vi "Module - Page User.vi"() -> ()   [LabVIEW 2020]
uses:
  Control/Cluster - User Information.ctl
  Control/Header - User Access Level.ctl
  Control/Button/Select Option 2.ctl
  Control/State - Module User Management.ctl
  Control/Password Setting Data.ctl
  Control/State - FGV.ctl
  Control/State - eFGV.ctl
  Control/aFGV States - Subpanel.ctl
  Control/User Authorization Info.ctl
  Control/Header - User Management.ctl
  a4231f55-2fe4-47fd-8ff5-63e6bb856ac6.vi
  762b96f1-960b-474f-bf97-e387c57ec164.vi
  Control/State - Directory.ctl
panel:
  in  "Tab Control":T1(tab)
  in  "Filter:":string(combo)="Show All" caption="Select Access Level:"
  in  "Clear Search":bool
  in  "Search Bar":string
  in  "Search By:":T2
  in  "Setting":bool
  in  "Add User":bool
  in  "User Information":T3[](array[typedef])
  in  "Stop":bool
  out "Header":T4
  in  "Search User":string(combo)
  out "Delete Msg":bool
  in  "Config: Access Level":string(combo) caption="Access Level:"
  in  "Password:":string
  in  "Username:":string
  in  "Name:":string
  in  "Config: Update":bool
  in  "Back 1":bool
  in  "Config: All Page":i32(listbox) caption="All Page"
  in  "Config: Accessible Page":i32(listbox) caption="Accessible Page"
  in  "Config: Add Page":bool
  in  "Config: Delete Page":bool
  in  "Config: Reset Page":bool
  in  "Back 2":bool
  in  "Manage: Access Level":string(combo)="Admin" caption="Access Level:"
  in  "Manage: All Page":i32(listbox) caption="All Page"
  in  "Manage: Accessible Page":i32(listbox) caption="Accessible Page"
  in  "Manage: Delete Page":bool
  in  "Manage: Add Page":bool
  in  "Header - User Access Level":T5
  in  "Staff Id":string caption="Staff Id:"
  in  "New Name:":string caption="Name:"
  in  "New Username:":string caption="Username:"
  in  "New Password:":string caption="Password:"
  in  "New Access Level:":string(combo) caption="Access Level:"
  in  "Re-Type Password:":string caption="Password:"
  in  "Create User":bool
  in  "Cancel Create User":bool
  in  "Back 3":bool
  in  "User Information T":i32(listbox) caption="User Information Listbox"
  in  "Access Page T":i32(listbox) caption="User Information Listbox"
  # "Manage User Account"
  # "Configure User Account"
  # "Manage User Access"
  # "Create New User"
  # "Fill up all information"
  # "Data Acquisition System"
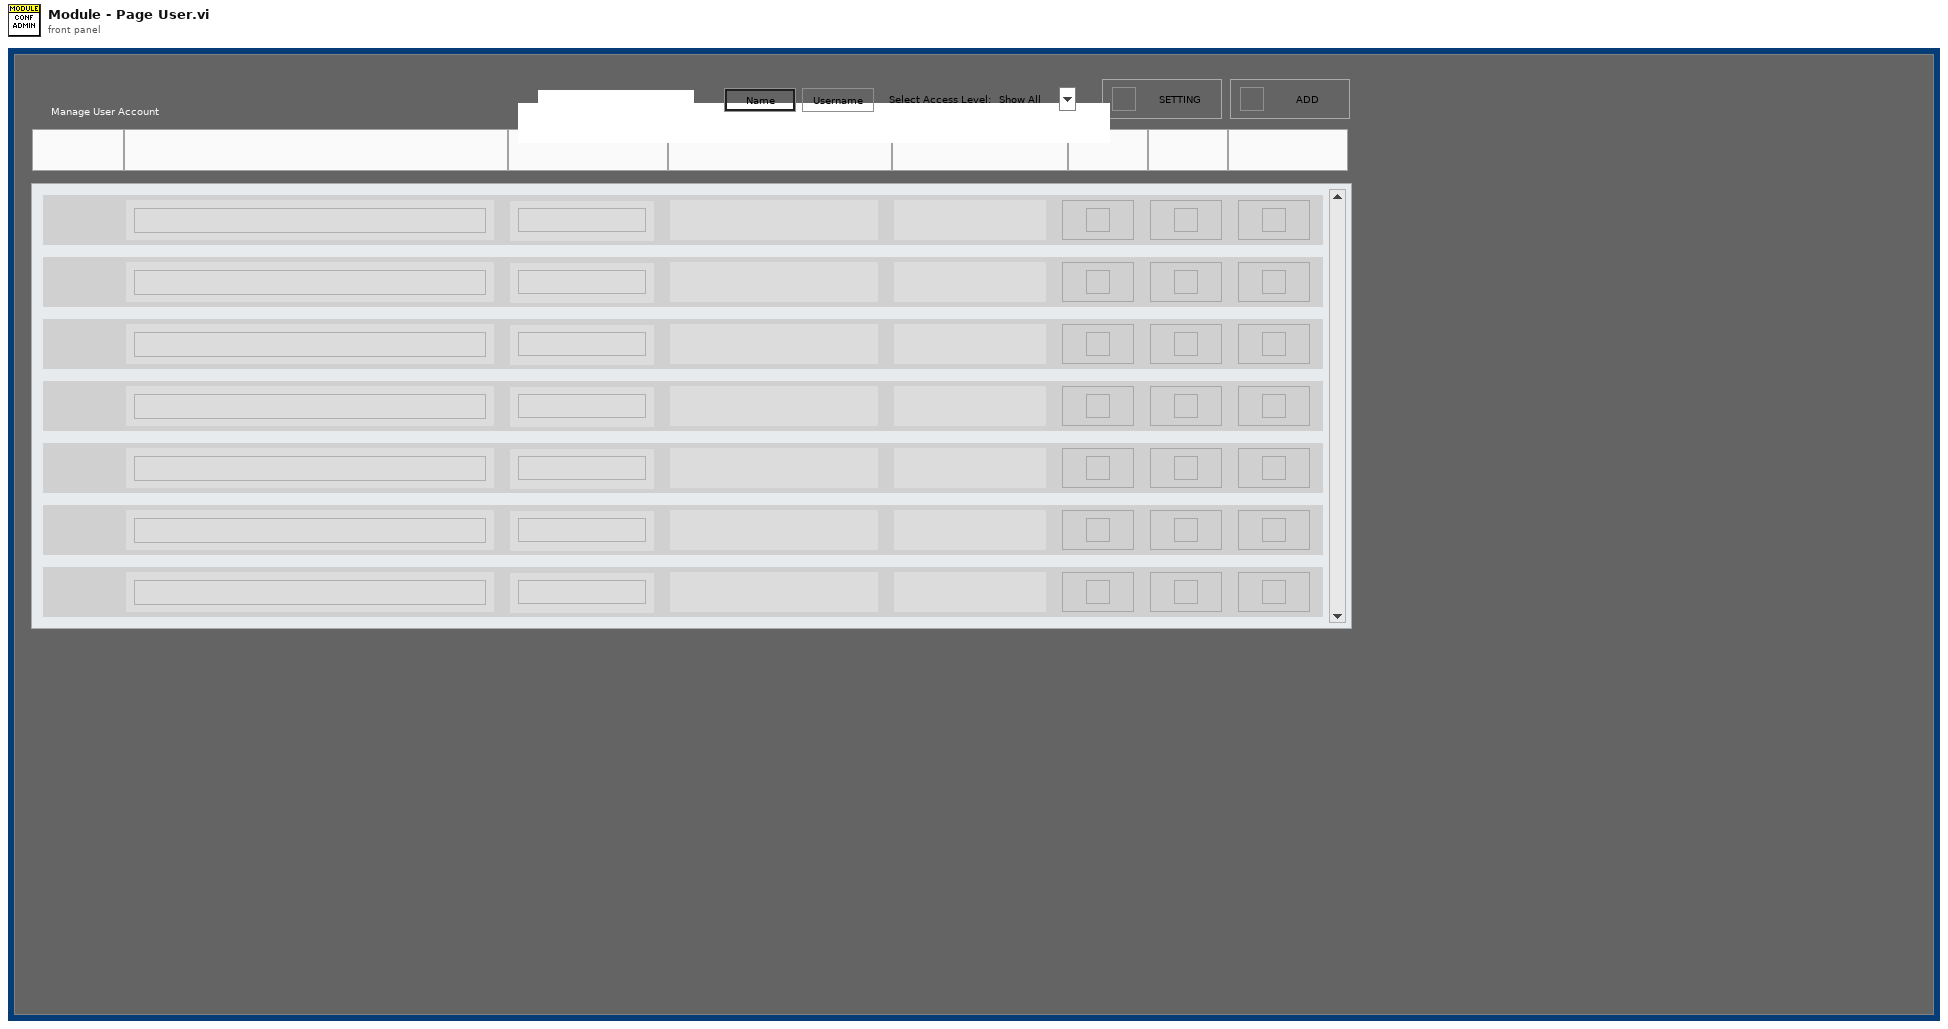
[diagram p1: front panel]
types:
  T1 = enum32{"Table", "Edit User", "Config", "New User", "Preference"}
  T2 = typedef "Select Option 2.ctl" = enum32{"L", "R"}
  T3 = typedef "Cluster - User Information.ctl" = cluster{"Access Level":u16, "Name":string, "Staff ID":string, "Username":string, "Password":string, "Configure":bool, "Status":bool, "Remove":bool}
  T4 = cluster{"Data 1":string, "Data 2":string, "Data 3":string, "Data 4":string, "Data 5":string, "Data 7":string, "Data 8":string, "Data 9":string}
  T5 = typedef "Header - User Access Level.ctl" = enum16{"Admin", "Manager", "Engineer", "Technician"}
  T6 = enum16{"Init", "Init Page", "Register Events", "Load User Access Page", "Load User Authorization Info", "Create Folder Data", "Update Folder Data", "Logout", "Idle", "Query DB Authrorization Info", "Update Authorization Info", "Reset User Access Page", "Add User Access Page", "Remove User Access Page", "Save User Authorization Info", "Search User", "Verify New User", "Create New User", "Update Authrorization Data", "Update Selected User", "Edit User Info", "Check Logged User", "Remove", "Block", "Add Config Access Page", "Remove Config Access Page", "Update Config User Access", "Save Config Access Page", "Save Password Settg", "Exit"}
  T7 = typedef "Password Setting Data.ctl" = cluster{"Length":i32, "Special Char":i32, "Numeric":i32, "Alphabet":i32}
  T8 = cluster{"Table":string[][], "Selected Row":i32, "Process":string, "Password Setting":T7, "Column Header Strings":string[], "Initialized Row":string[], "User Info":cluster{"Name":string, "Username":string, "Password":string, "Level":string, "Block":string, "Show Password":bool}, "Path User Info":path, "Path User Access":path, "Update User":bool, "Old Username":string, "Username Updated?":bool, "User Information":cluster{"All":T3[], "Filtered":T3[]}}
  T9 = typedef "State - Module User Management.ctl" = enum16{"Init", "Init Page", "Register Events", "Load User Access Page", "Load User Authorization Info", "Create Folder Data", "Update Folder Data", "Logout", "Idle", "Query DB Authrorization Info", "Update Authorization Info", "Reset User Access Page", "Add User Access Page", "Remove User Access Page", "Save User Authorization Info", "Search User", "Verify New User", "Create New User", "Update Authrorization Data", "Update Selected User", "Edit User Info", "Check Logged User", "Remove", "Block", "Add Config Access Page", "Remove Config Access Page", "Update Config User Access", "Save Config Access Page", "Save Password Settg", "Exit"}
  T10 = typedef "State - FGV.ctl" = enum16{"Write", "Read"}
  T11 = typedef "aFGV States - Subpanel.ctl" = enum16{"Init", "Get VI Name", "Update", "Exit"}
  T12 = typedef "State - eFGV.ctl" = enum16{"Init", "Read", "Write", "Exit"}
  T13 = typedef "Header - User Management.ctl" = enum16{"Name", "Staff ID", "Username", "Password", "Access Level", "Status", "Access Page"}
  T14 = enum8{"Enabled", "Disabled", "Disabled and Grayed Out"}
  T15 = enum32{"Table", "Edit User", "Config", "New User"}
  T16 = typedef "State - Directory.ctl" = enum16{"Plant", "Config", "Admin", "Password", "Modules", "Dialog Box", "SubVI", "Setting"}
  T17 = enum16{"open", "replace", "create", "open or create", "replace or create", "replace or create with confirmation"}
  T18 = typedef "Page List Configuration.ctl" = cluster{"HMI Configuration":cluster{"EXE Name":string, "Project Name":string, "Max Page No":i32, "HMI State":enum32{"Invalid", "Standard", "Closed", "Hidden", "Minimized", "Maximized"}, "Version":enum16{"Demo", "User"}, "Check License":bool, "Font Size":u32, "Res: Height":i16, "Res: Width":i16, "License Level":enum16{"Level 1", "Level 2", "Level 3", "Level 4", "Level 5"}, "License Type":enum16{"Free", "Trial", "Subscription", "Perpetual"}}, "All HMI Module":string[], "Default HMI Module":string[], "Page Module":string[], "Page List: Level 1":string[], "Page List: Level 2":string[], "Page List: Level 3":string[], "All RT Module":string[], "Default RT Module":string[], "Acquire Enable Page":string[], "Log Enable Page":string[], "Run Page":string[], "Kill Page":string[], "Button":cluster{"Text":string[], "Tip Strip":string[]}}
  T19 = typedef "License File Parameter.ctl" = cluster{"Expired Time":string, "Computer ID":string, "Product Name":string, "Period":i16, "Activated Time":string, "License Level":enum16{"Level 1", "Level 2", "Level 3", "Level 4", "Level 5"}, "License Type":enum16{"Free", "Trial", "Subscription", "Perpetual"}, "Log Time":string}
  T20 = enum16{"Level 1", "Level 2", "Level 3", "Level 4", "Level 5"}
  T21 = cluster{"Access Level:":string, "List Page":string[]}[]
  T22 = typedef "User Authorization Info.ctl" = cluster{"Name":string, "Username":string, "Password":string, "Access Level:":string, "Block":string, "List Page":string[]}
  T23 = cluster{"Access Level":bool, "Name":bool, "Staff ID":bool, "Username":bool, "Password":bool, "Configure":bool, "Status":bool, "Remove":bool}
  T24 = enum32{"invalid app kind", "Development System", "Run Time System", "Student Edition", "Embedded LabVIEW", "Evaluation", "Custom"}
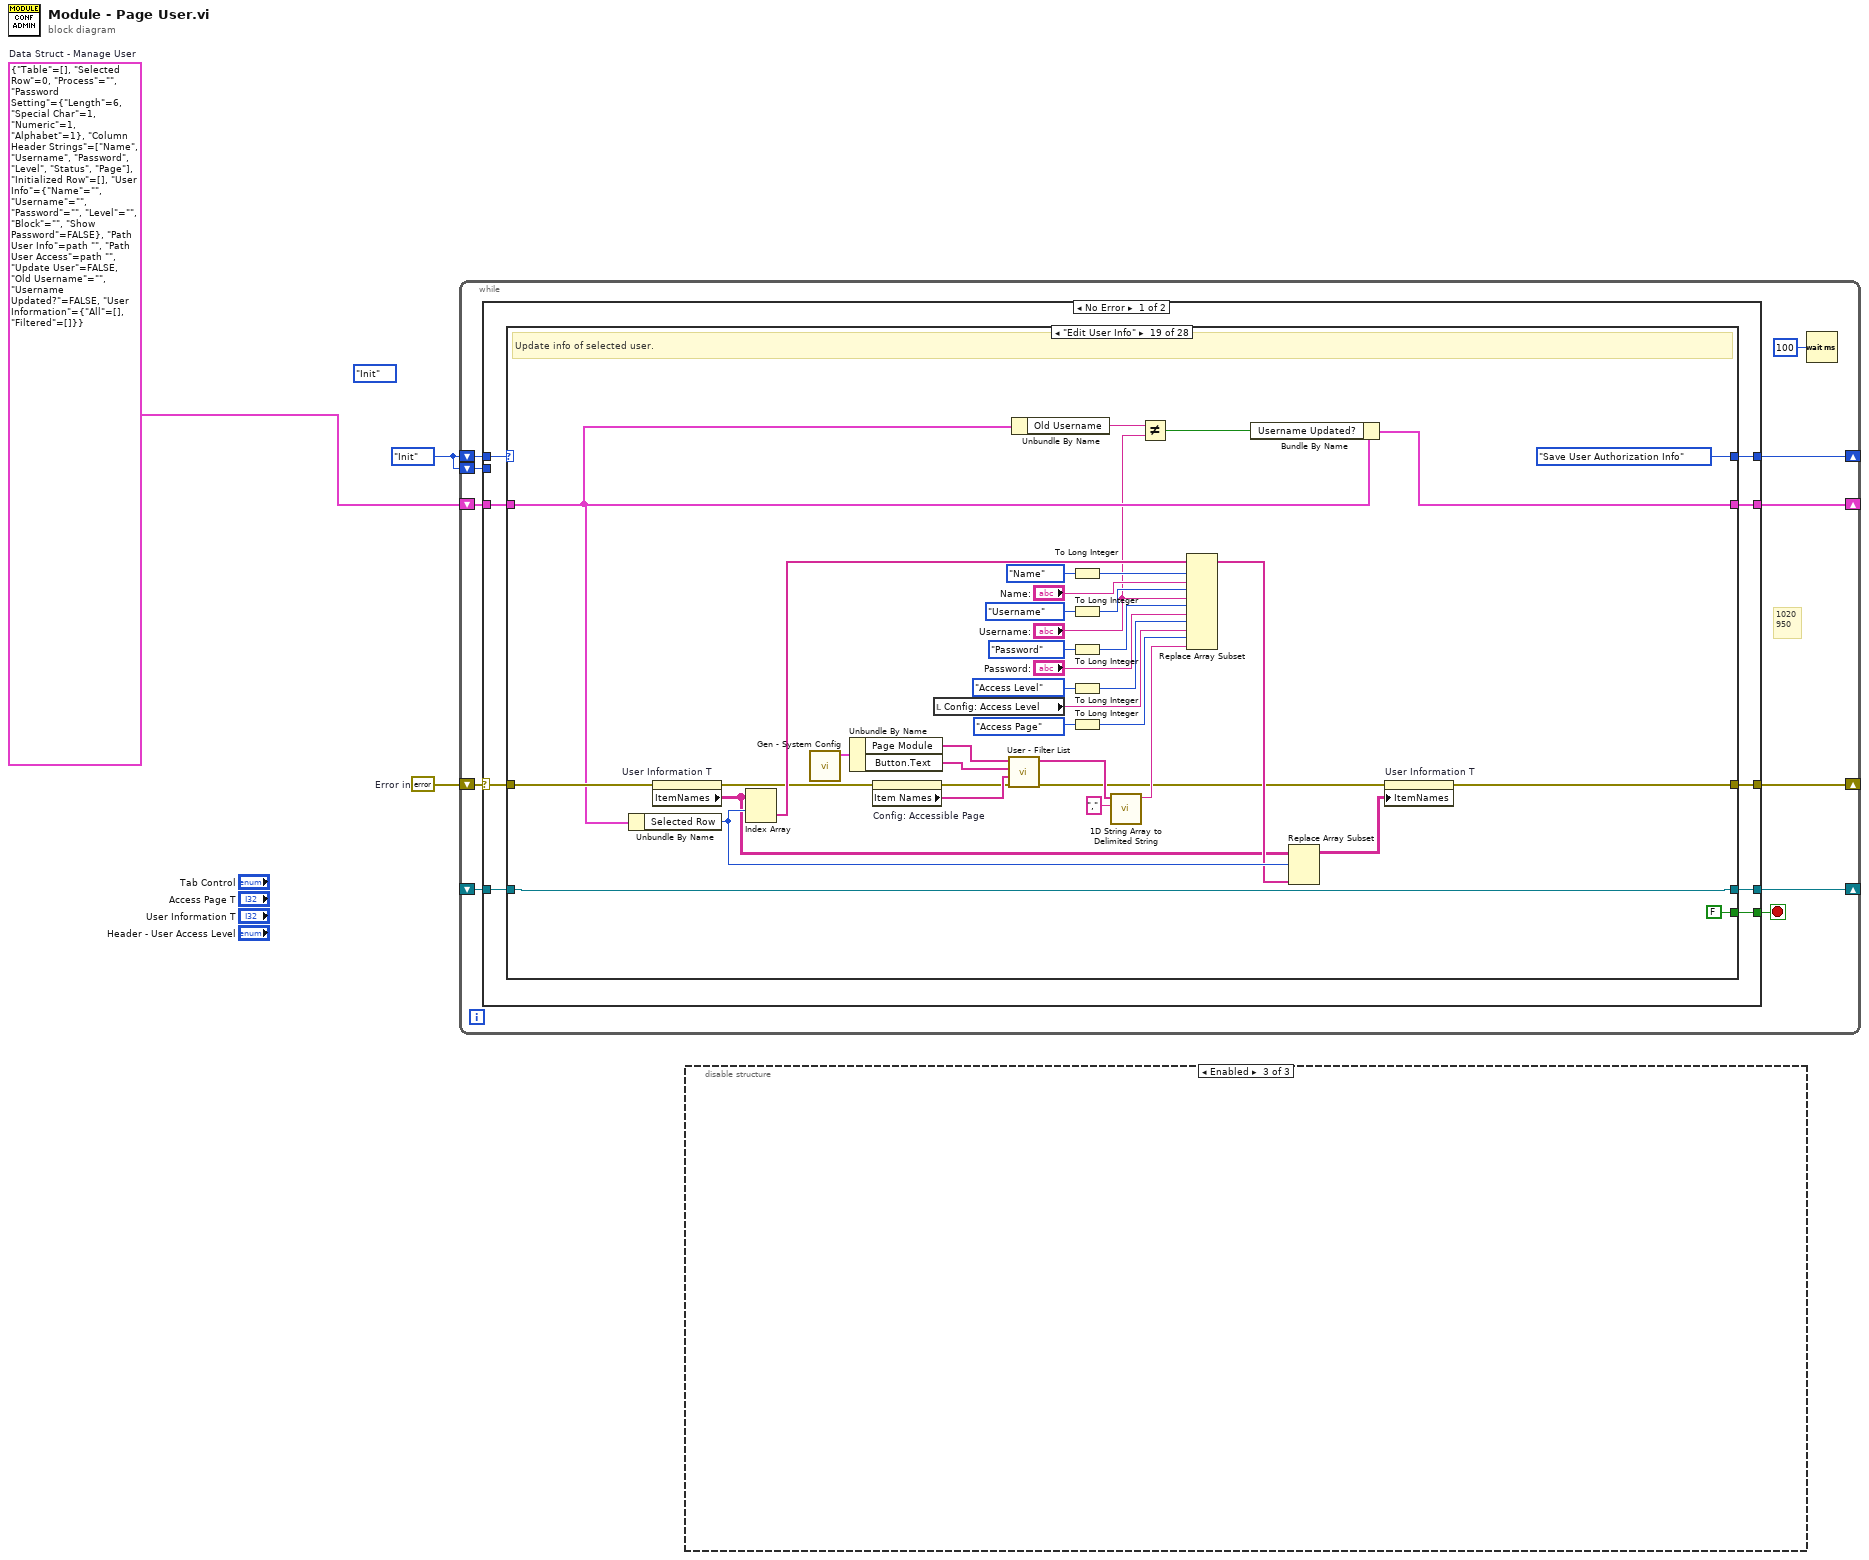
[diagram p0: block diagram]
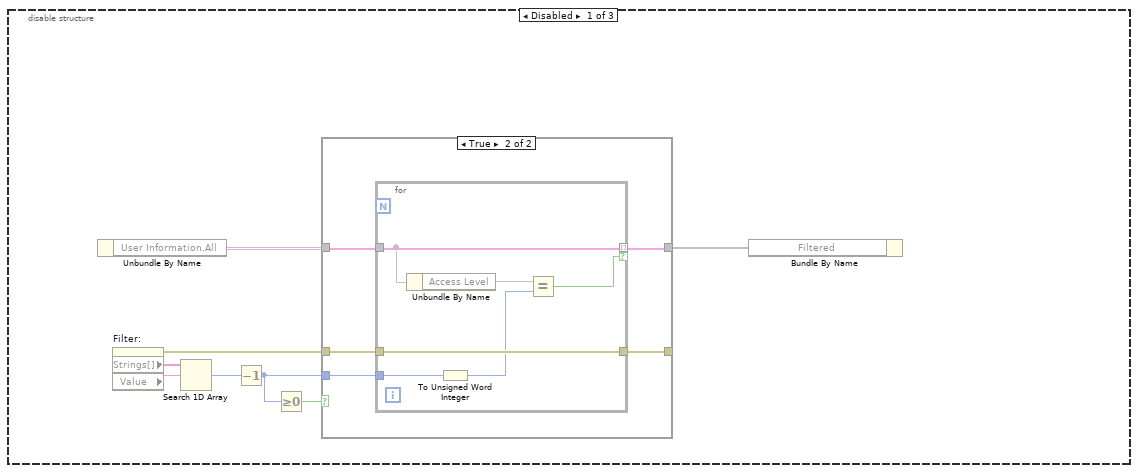
[diagram p2: hidden frame]
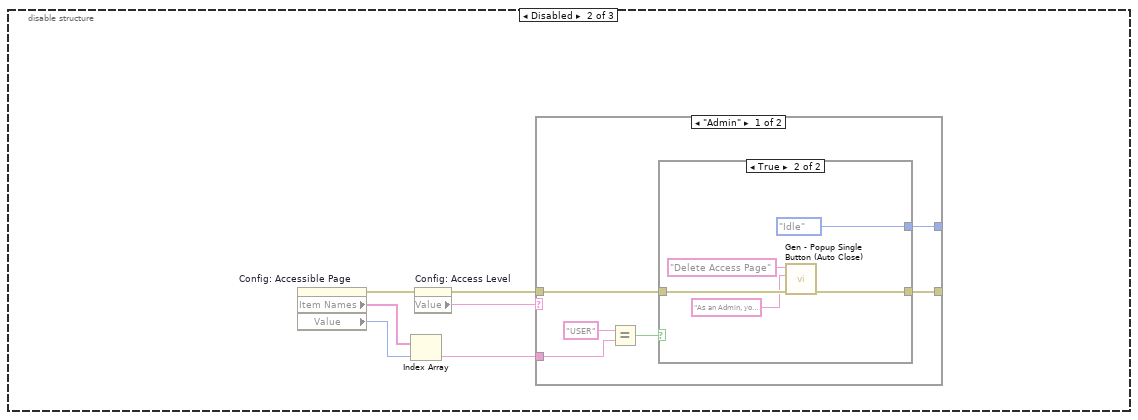
[diagram p4: hidden frame]
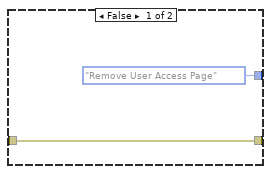
[diagram p5: hidden frame]
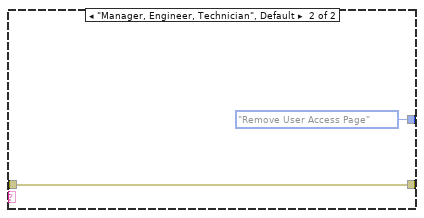
[diagram p6: hidden frame]
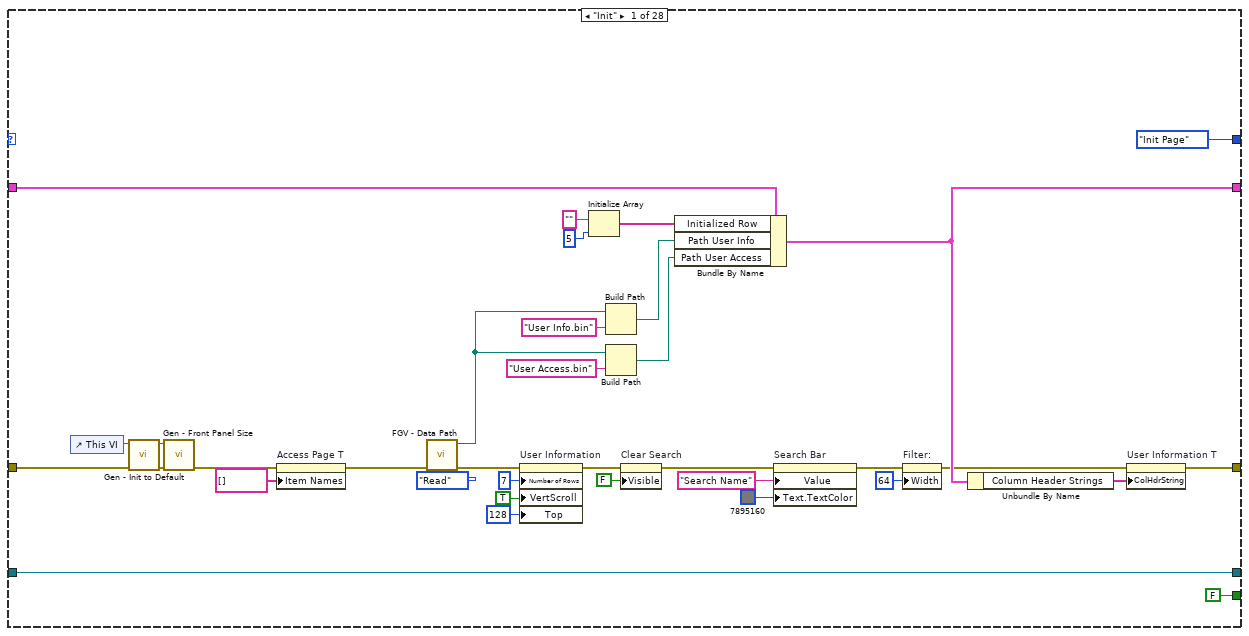
[diagram p7: hidden frame]
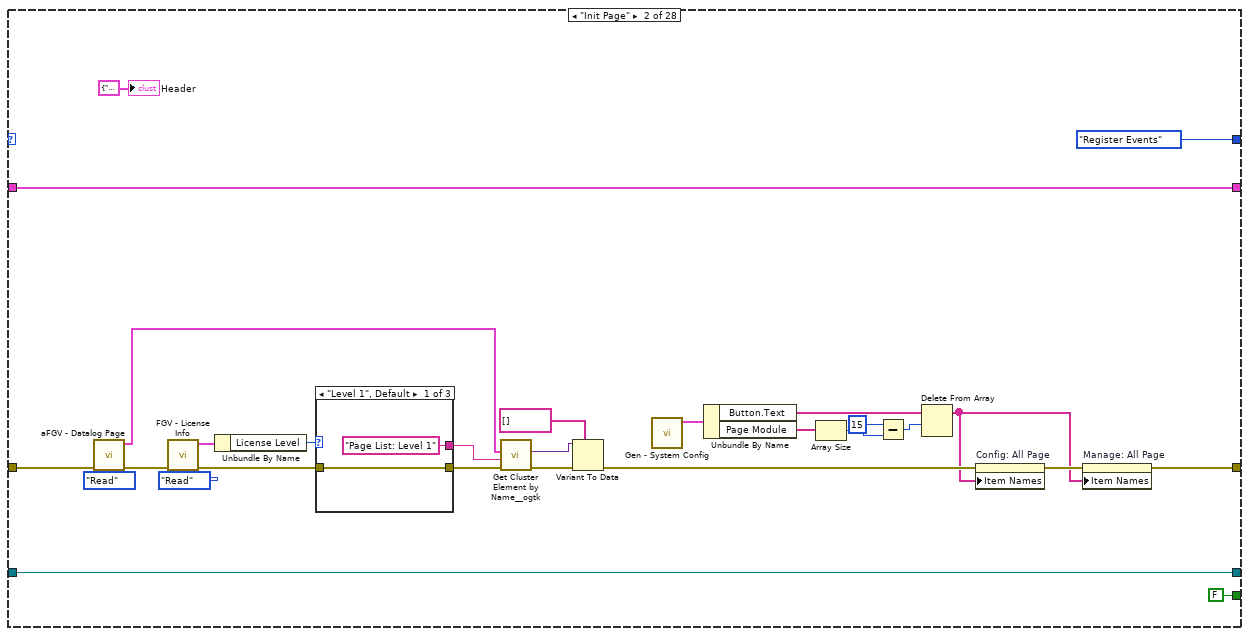
[diagram p8: hidden frame]
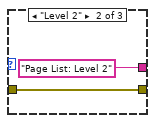
[diagram p9: hidden frame]
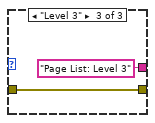
[diagram p10: hidden frame]
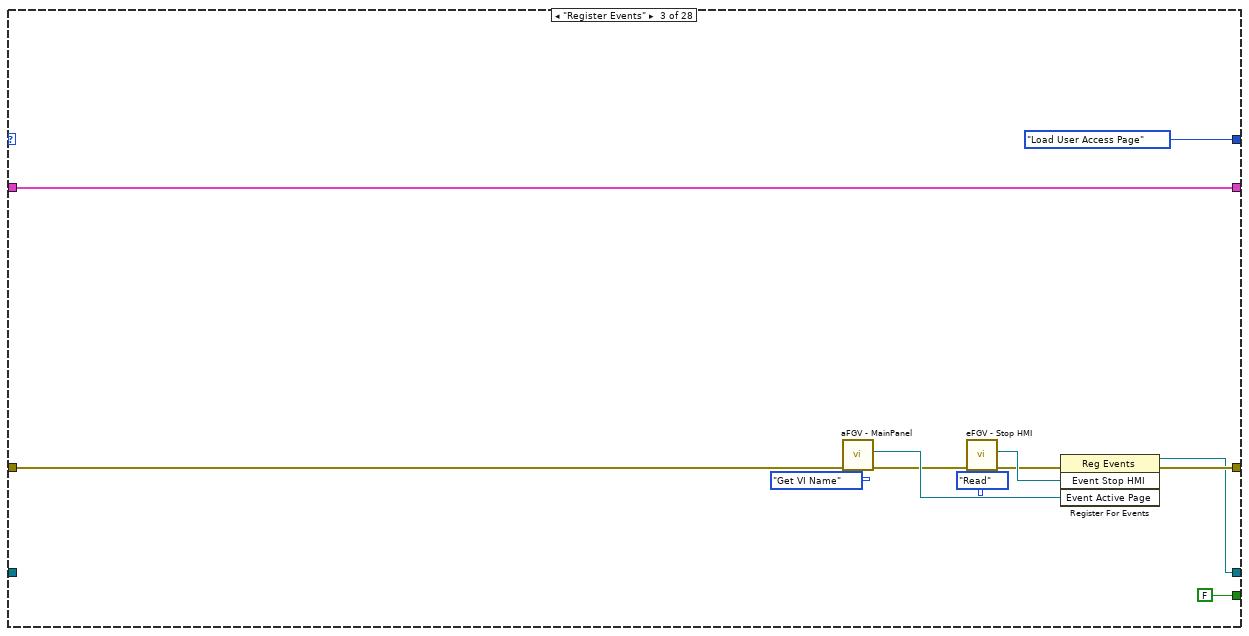
[diagram p11: hidden frame]
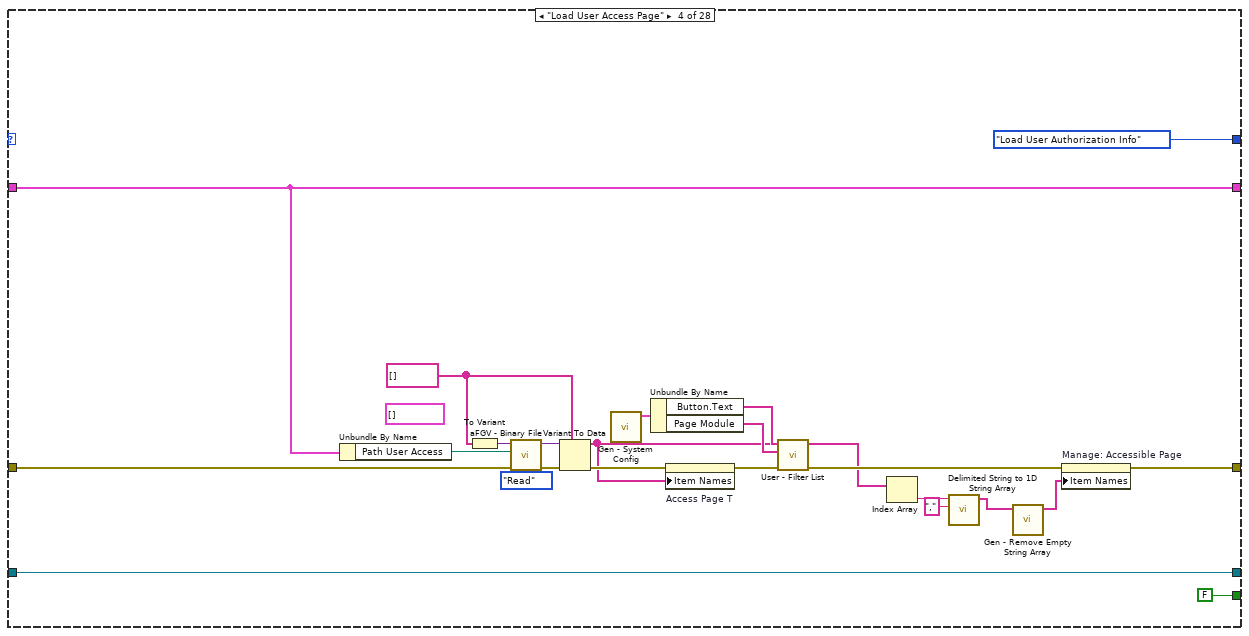
[diagram p12: hidden frame]
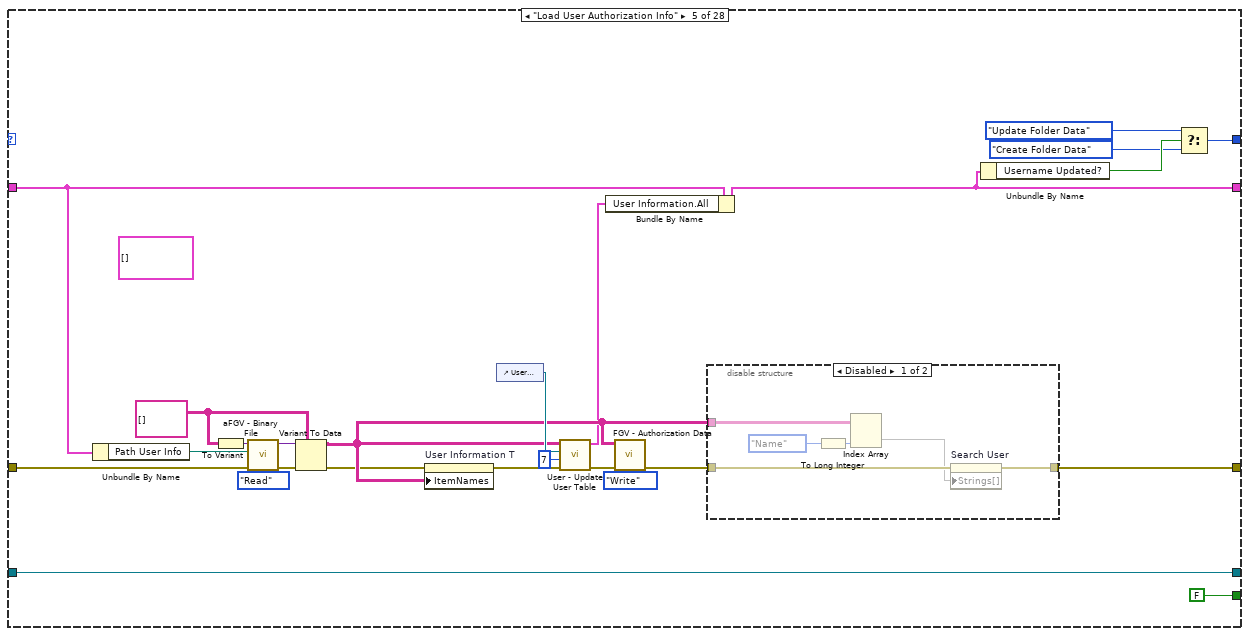
[diagram p13: hidden frame]
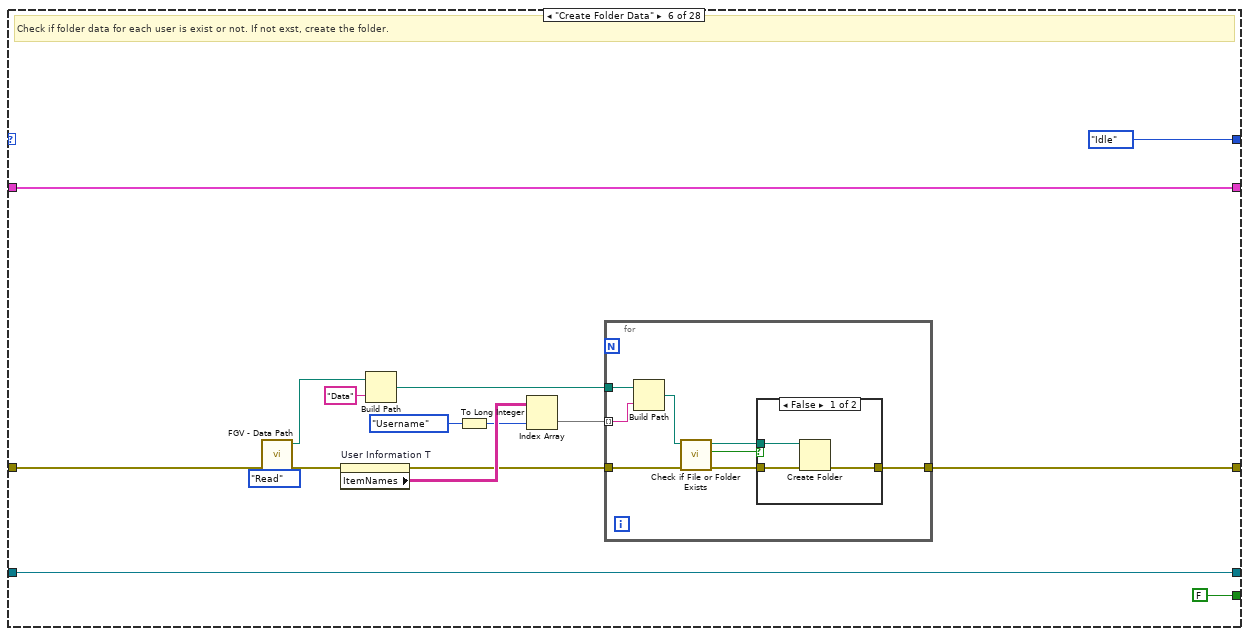
[diagram p15: hidden frame]
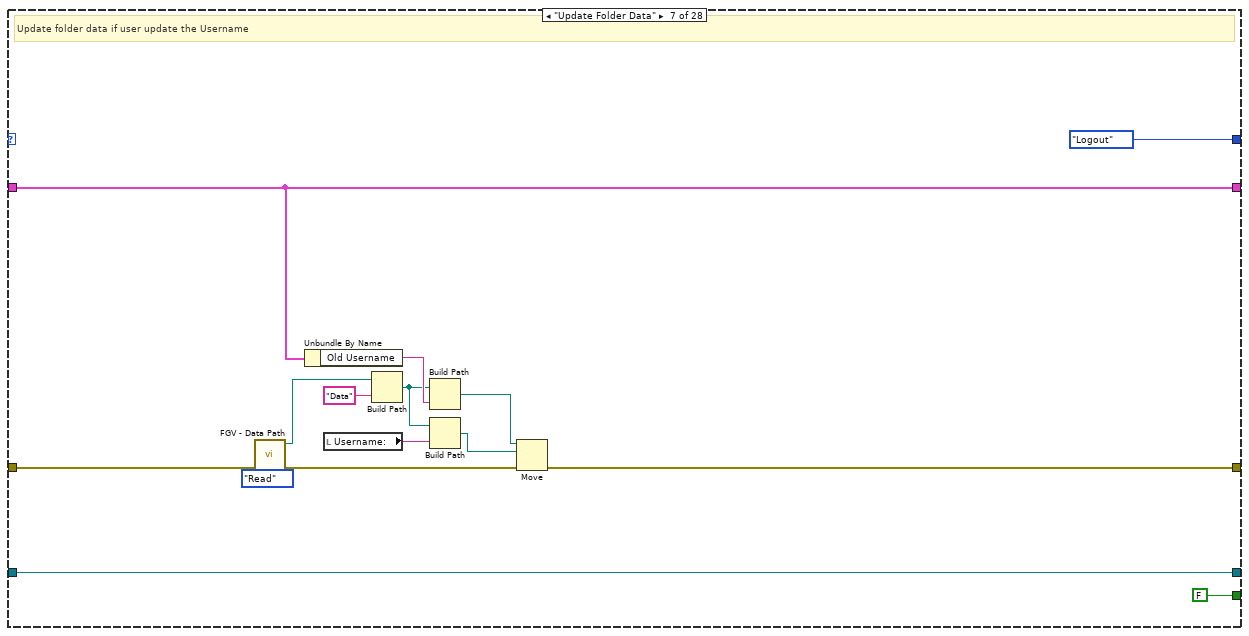
[diagram p17: hidden frame]
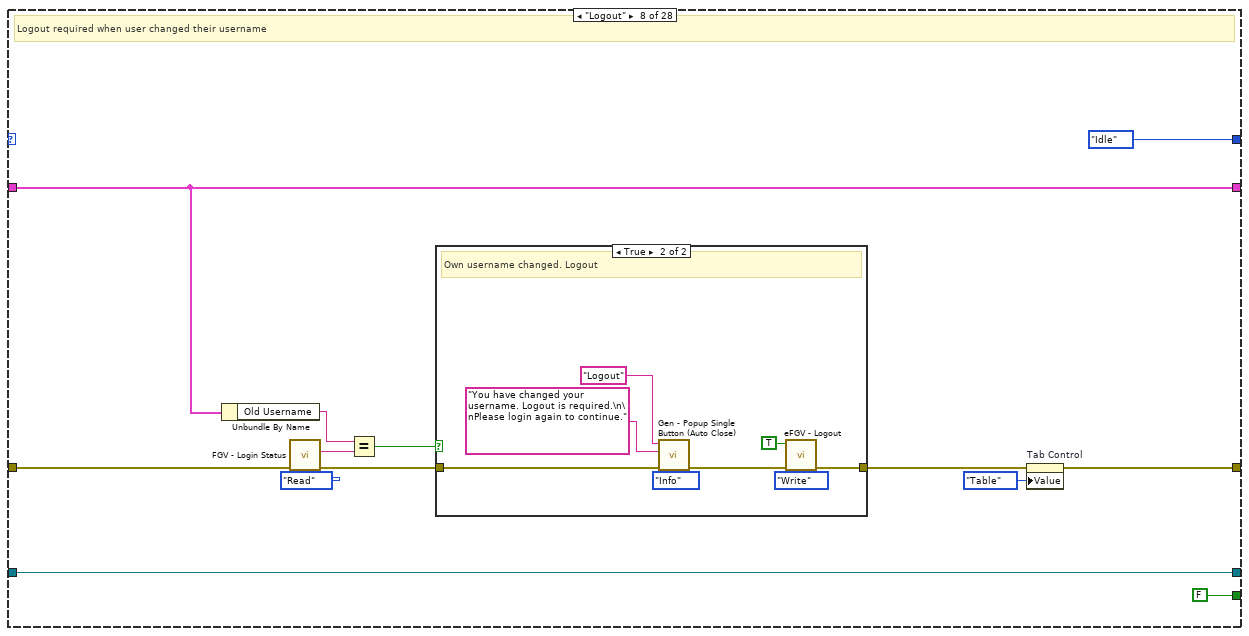
[diagram p18: hidden frame]
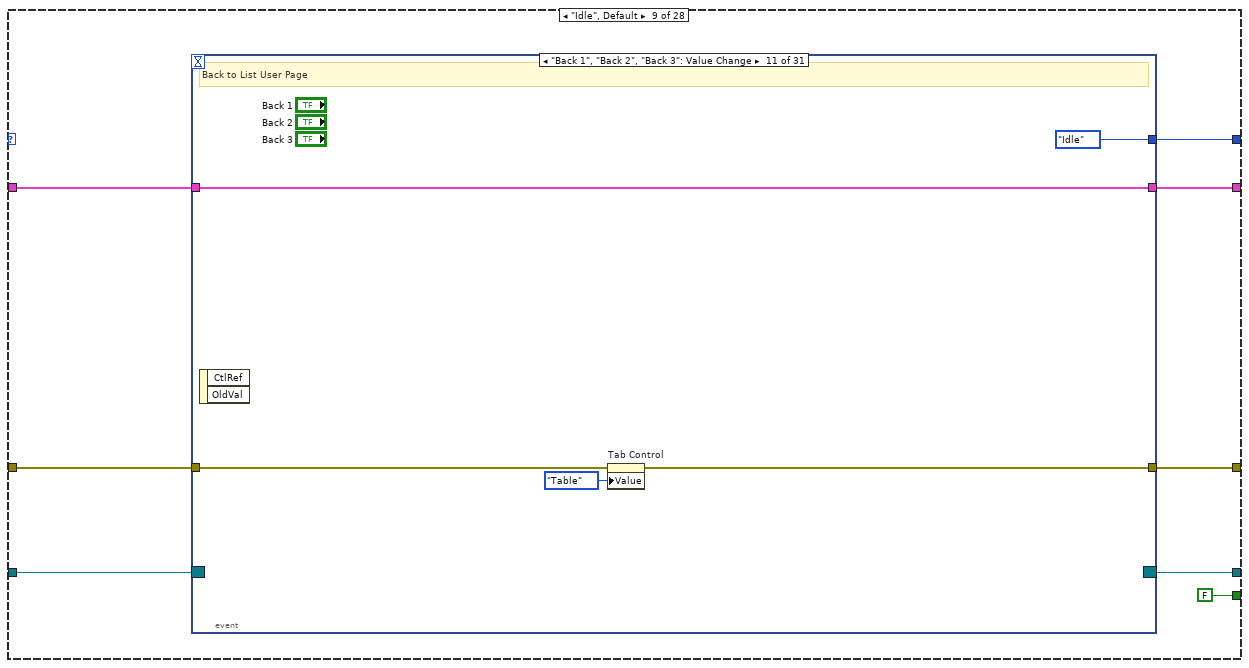
[diagram p20: hidden frame]
diagram:
  (unwired) T6."Init"
  w2 = T8 {"Table"=[], "Selected Row"=0, "Process"="", "Password Setting"={"Length"=6, "Special Char"=1, "Numeric"=1, "Alphabet"=1}, "Column Header Strings"=["Name", "Username", "Password", "Level", "Status", "Page"], "Initialized Row"=[], "User Info"={"Name"="", "Username"="", "Password"="", "Level"="", "Block"="", "Show Password"=FALSE}, "Path User Info"=path "", "Path User Access"=path "", "Update User"=FALSE, "Old Username"="", "Username Updated?"=FALSE, "User Information"={"All"=[], "Filtered"=[]}}  # Data Struct - Manage User
  w1 = State_-_Module_User_Management."Init"
  w3 = errorcluster {"status"=FALSE, "code"=0, "source"=""}  # Error in
  n1 = while {
    shift-right: [w12] -> _
    shift-left: w3 -> [w14]
    shift-right: [w6] -> _
    shift-left: w1 -> [w13]
    shift-right: [w9] -> _
    shift-left: w2 -> [w11]
    shift-right: [w8] -> _
    shift-left: _ -> [w7]
    shift-left: w1 -> [w4]
    stop <- w10 stop-if-true
    # "1020\n950"
    n2 = case shown="No Error" w14 {
      selector: w14 -> [w22 w1073]
      tunnel: w13 -> [w23 _]
      tunnel: [w21 w1072] -> w12
      tunnel: w11 -> [w20 w1079]
      tunnel: [w19 FALSE] -> w10
      tunnel: [w18 w1079] -> w9
      tunnel: [w17 w1078] -> w8
      tunnel: w7 -> [w16 w1078]
      tunnel: [w15 State_-_Module_User_Management."Idle"] -> w6
      tunnel: w4 -> [_ w1071]
      frame No Error {
        n3 = case shown="\"Edit User Info\"" w23 {
          tunnel: [w55 w70 w102 w121 w152 w164 w188 w204 w231 w555 w584 w616 w635 w663 w685 w726 w766 w781 w823 w847 w876 w908 w933 w963 w1000 w1007 w1024 w1067] -> w21
          tunnel: w22 -> [w46 w74 w95 w122 w142 w171 w198 w209 w232 w568 w601 w608 w641 w664 w711 w748 w762 w801 w839 w856 w875 w905 w941 w971 w995 w1006 w1020 w1070]
          tunnel: w20 -> [w52 w85 w103 w125 w134 w169 w195 w212 w230 w572 w602 w627 w638 w662 w714 w751 w770 w800 w811 w857 w877 w914 w951 w977 w1004 w1005 w1016 w1068]
          tunnel: [FALSE FALSE FALSE FALSE FALSE FALSE FALSE FALSE FALSE FALSE FALSE FALSE FALSE FALSE FALSE FALSE FALSE FALSE FALSE FALSE FALSE FALSE FALSE FALSE FALSE FALSE FALSE TRUE] -> w19
          tunnel: [w38 w85 w103 w125 w129 w169 w195 w212 w229 w572 w602 w627 w638 w662 w714 w751 w770 w774 w809 w857 w877 w913 w951 w977 w1004 w1005 w1016 w1068] -> w18
          tunnel: [w57 w84 w99 w124 w151 w175 w202 w215 w228 w575 w605 w630 w644 w667 w713 w750 w769 w804 w842 w859 w879 w918 w950 w976 w1003 w1015 w1023 w1066] -> w17
          tunnel: w16 -> [w57 w84 _ w124 w151 w175 w202 w215 w227 w575 w605 w630 w644 w667 w713 w750 w769 w804 w842 w859 w879 w918 w950 w976 w1003 w1015 w1023 w1066]
          tunnel: [State_-_Module_User_Management."Init Page" State_-_Module_User_Management."Register Events" State_-_Module_User_Management."Load User Access Page" State_-_Module_User_Management."Load User Authorization Info" w130 State_-_Module_User_Management."Idle" State_-_Module_User_Management."Logout" State_-_Module_User_Management."Idle" w225 State_-_Module_User_Management."Edit User Info" State_-_Module_User_Management."Save User Authorization Info" State_-_Module_User_Management."Save User Authorization Info" State_-_Module_User_Management."Load User Authorization Info" State_-_Module_User_Management."Idle" w683 State_-_Module_User_Management."Save User Authorization Info" State_-_Module_User_Management."Idle" State_-_Module_User_Management."Idle" State_-_Module_User_Management."Save User Authorization Info" w844 w870 State_-_Module_User_Management."Save User Authorization Info" State_-_Module_User_Management."Save Config Access Page" State_-_Module_User_Management."Save Config Access Page" State_-_Module_User_Management."Save Config Access Page" State_-_Module_User_Management."Idle" State_-_Module_User_Management."Idle" State_-_Module_User_Management."Exit"] -> w15
          frame "Init" {
            n4 = control-ref of="This VI"() -> (w47:refnum<vi>)
            n5 = call "Gen - Init to Default.vi"("Error in"=w46, "This VI"=w47) -> ("Error out"=w48:errorcluster)  [unwired: 8 in, 1 out]
            n6 = call "Gen - Front Panel Size.vi"("Error In"=w48, "This VI"=w47) -> ("Error Out"=w37:errorcluster)  [unwired: 9 in]
            n7 = property on="Access Page T" class="LstBox (strict)"(error in=w37, "Item Names"=string[] []) -> (error out=w36:errorcluster)  [unwired: 1 in, 1 out]
            n8 = call "FGV - Data Path.vi"("FGV State"=State_-_FGV."Read", "Error In"=w36) -> ("Error Out"=w40:errorcluster, "Path Out"=w32:path)  [unwired: 8 in]
            n9 = property on="User Information" class="Arr"(error in=w40, "Number of Rows"=u32 7, "VertScroll"=TRUE ("Vertical Scrollbar Visible"), "Top"=128 ("Position:Top")) -> (error out=w31:errorcluster)  [unwired: 1 in, 1 out]
            n10 = Initialize Array("", 5 ("dimension size")) -> (w49:string[])
            n11 = Build Path(base path=w32, name or relative path="User Info.bin") -> (appended path=w42:path)
            n12 = Build Path(base path=w32, name or relative path="User Access.bin") -> (appended path=w41:path)
            n13 = property on="Clear Search" class="Bool"(error in=w31, "Visible"=FALSE) -> (error out=w27:errorcluster)  [unwired: 1 in, 1 out]
            n14 = Bundle By Name(cluster=w52, "Initialized Row"=w49, "Path User Info"=w42, "Path User Access"=w41) -> (w38:T8)
            n15 = property on="Search Bar" class="Str"(error in=w27, "Value"="Search Name" ("Search Bar"), "Text.TextColor"=u32 7895160) -> (error out=w26:errorcluster)  [unwired: 1 in, 1 out]
            n16 = property on="Filter:" class="CmbBox"(error in=w26, "Width"=u32 64 ("Size:Width")) -> (error out=w25:errorcluster)  [unwired: 1 in, 1 out]
            n17 = Unbundle By Name(w38) -> ("Column Header Strings"=w53:string[])
            n18 = property on="User Information T" class="MCListbox (strict)"(error in=w25, "ColHdrString"=w53) -> (error out=w55:errorcluster)  [unwired: 1 in, 1 out]
          }
          frame "Init Page" {
            n19 = call "aFGV - Datalog Page.vi"("Action"=enum16{"Read", "Write"}."Read", "Error In"=w74) -> ("Error Out"=w79:errorcluster, "Data Out"=w73:T18)  [unwired: 8 in]
            n20 = call "FGV - License Info.vi"("FGV States"=enum16{"Read", "Write"}."Read", "Error In"=w79) -> ("Error Out"=w66:errorcluster, "License Info"=w77:T19)  [unwired: 8 in]
            n21 = Unbundle By Name(w77) -> ("License Level"=w69:T20)
            n22 = case shown="\"Level 1\", Default" w69 {
              tunnel: ["Page List: Level 1" "Page List: Level 2" "Page List: Level 3"] -> w68
              tunnel: [w87 w88 w90] -> w67
              tunnel: w66 -> [w87 w88 w90]
              frame "Level 1", Default {
              }
              frame "Level 2" {
              }
              frame "Level 3" {
              }
            }
            n23 = call <userlib>:"Get Cluster Element by Name__ogtk.vi"("error in (no error)"=w67, "Element Name"=w68, "Cluster"=w73) -> ("error out"=w80:errorcluster, "VElement"=w82:variant)  [unwired: 6 in, 1 out]
            n24 = Variant To Data(error in=w80, type=string[] [], Variant=w82) -> (error out=w72:errorcluster)  [unwired: 1 out]
            n25 = call "Gen - System Config.vi"() -> ("Data Out"=w65:T18)  [unwired: 11 in]
            n26 = Unbundle By Name(w65) -> ("Button.Text"=w60:string[], "Page Module"=w63:string[])
            n27 = Array Size(array=w63) -> (size(s)=w64:i32)
            n28 = Subtract(x=15, y=w64) -> (x-y=w61:i32)
            n29 = Delete From Array(array=w60, length=w61) -> (array with subset deleted=w62:string[])  [unwired: 1 in, 1 out]
            n30 = property on="Config: All Page" class="LstBox (strict)"(error in=w72, "Item Names"=w62) -> (error out=w71:errorcluster)  [unwired: 1 in, 1 out]
            n31 = property on="Manage: All Page" class="LstBox (strict)"(error in=w71, "Item Names"=w62) -> (error out=w70:errorcluster)  [unwired: 1 in, 1 out]
            "Header" <- T4 {"Data 1"="Level", "Data 2"="Name", "Data 3"="Staff ID", "Data 4"="Username", "Data 5"="Password", "Data 7"="Info", "Data 8"="Status", "Data 9"="Remove"} ("Header")
          }
          frame "Register Events" {
            n32 = call "aFGV - MainPanel.vi"("Action"=aFGV_States_-_Subpanel."Get VI Name", "Error In"=w95) -> ("Error Out"=w93:errorcluster, "Event Active Page"=w96:refnum<user-event>)  [unwired: 7 in, 1 out]
            n33 = call "eFGV - Stop HMI.vi"("Action"=State_-_eFGV."Read", "Error In"=w93) -> ("Error Out"=w100:errorcluster, "Event Stop HMI"=w101:refnum<user-event>)  [unwired: 7 in, 1 out]
            n34 = register-events(error in=w100, w101, w96) -> (reference out=w99:refnum<event-registration>, error out=w102:errorcluster)  [unwired: 1 in]
          }
          frame "Load User Access Page" {
            w116 = string[] []
            (unwired) T21 []
            n35 = Unbundle By Name(w125) -> ("Path User Access"=w120:path)
            n36 = To Variant(anything=w116) -> (Variant=w118:variant)
            n37 = call "aFGV - Binary File.vi"("State"=enum16{"Read", "Write"}."Read", "Error In"=w122, "Path"=w120, "Data in"=w118) -> ("Error Out"=w113:errorcluster, "Data Out"=w119:variant)  [unwired: 6 in]
            n38 = Variant To Data(error in=w113, type=w116, Variant=w119) -> (data=w107:string[], error out=w117:errorcluster)
            n39 = call "Gen - System Config.vi"() -> ("Data Out"=w112:T18)  [unwired: 11 in]
            n40 = Unbundle By Name(w112) -> ("Button.Text"=w110:string[], "Page Module"=w111:string[])
            n41 = property on="Access Page T" class="LstBox (strict)"(error in=w117, "Item Names"=w107) -> (error out=w109:errorcluster)  [unwired: 1 in, 1 out]
            n42 = call "User - Filter List.vi"("Error In"=w109, "Data to Search"=w107, "Search From"=w111, "All List"=w110) -> ("Error Out"=w108:errorcluster, "Data Out"=w106:string[])  [unwired: 6 in]
            n43 = Index Array(array=w106) -> (element=w115:string)  [unwired: 1 in]
            n44 = call <vilib>:"Delimited String to 1D String Array.vi"("delimiter"=",", "delimited string"=w115) -> ("string array"=w105:string[])  [unwired: 9 in]
            n45 = call "Gen - Remove Empty String Array.vi"("Data Array"=w105) -> ("Data Out"=w104:string[])  [unwired: 10 in]
            n46 = property on="Manage: Accessible Page" class="LstBox (strict)"(error in=w108, "Item Names"=w104) -> (error out=w121:errorcluster)  [unwired: 1 in, 1 out]
          }
          frame "Load User Authorization Info" {
            w140 = string[][] []
            (unwired) T22[] []
            n47 = Unbundle By Name(w134) -> ("Path User Info"=w141:path)
            n48 = To Variant(anything=w140) -> (Variant=w136:variant)
            n49 = call "aFGV - Binary File.vi"("State"=enum16{"Read", "Write"}."Read", "Error In"=w142, "Path"=w141, "Data in"=w136) -> ("Error Out"=w137:errorcluster, "Data Out"=w143:variant)  [unwired: 6 in]
            n50 = Variant To Data(error in=w137, type=w140, Variant=w143) -> (data=w139:string[][], error out=w138:errorcluster)
            n51 = property on="User Information T" class="MCListbox (strict)"(error in=w138, "ItemNames"=w139) -> (error out=w148:errorcluster)  [unwired: 1 in, 1 out]
            n52 = control-ref of="User Information"() -> (w146:refnum<vi>)
            n53 = call "User - Update User Table.vi"("Error In"=w148, "Max visible row"=7, "User Infor Ref"=w146, "User Information"=w139) -> ("Error Out"=w147:errorcluster, "User Information Out"=w128:T3[])  [unwired: 6 in]
            n54 = Bundle By Name(cluster=w134, "User Information.All"=w128) -> (w129:T8)
            n55 = call "FGV - Authorization Data.vi"("State - FGV"=State_-_FGV."Write", "Error In"=w147, "Data In"=w139) -> ("Error Out"=w145:errorcluster)  [unwired: 7 in, 1 out]
            n56 = disable-structure shown="Disabled" {
              disable-tunnel: [w158 w159] -> w152
              disable-tunnel: w145 -> [w157 w159]
              disable-tunnel: w139 -> [w153 _]
              frame Disabled {
                n57 = To Long Integer(number=Header_-_User_Management."Name" ("Header - User Management")) -> (32bit integer=w154:i32)
                n58 = Index Array(array=w153, index (col)=w154) -> (element=w155:string[])  [unwired: 1 in]
                n59 = property on="Search User" class="CmbBox"(error in=w157, "Strings[]"=w155) -> (error out=w158:errorcluster)  [unwired: 1 in, 1 out]
              }
              frame Enabled {
              }
            }
            n60 = Unbundle By Name(w129) -> ("Username Updated?"=w133:bool)
            n61 = Select(t=State_-_Module_User_Management."Update Folder Data", s=w133, f=State_-_Module_User_Management."Create Folder Data") -> (s? t:f=w130:T9)
          }
          frame "Create Folder Data" {
            # "Check if folder data for each user is exist or not. If not exst, create the folder."
            n62 = call "FGV - Data Path.vi"("FGV State"=State_-_FGV."Read", "Error In"=w171) -> ("Error Out"=w168:errorcluster, "Path Out"=w161:path)  [unwired: 8 in]
            n63 = property on="User Information T" class="MCListbox (strict)"(error in=w168) -> (error out=w163:errorcluster, "ItemNames"=w167:string[][])  [unwired: 1 in, 1 out]
            n64 = Build Path(base path=w161, name or relative path="Data") -> (appended path=w160:path)
            n65 = To Long Integer(number=Header_-_User_Management."Username" ("Header - User Management")) -> (32bit integer=w165:i32)
            n66 = Index Array(array=w167, index (col)=w165) -> (element=w162:string[])  [unwired: 1 in]
            n67 = for {
              tunnel: [w178] -> w164
              tunnel: w163 -> [w183]
              tunnel: w162 -> [w181] mode=indexing
              tunnel: w160 -> [w182]
              n68 = Build Path(base path=w182, name or relative path=w181) -> (appended path=w180:path)
              n69 = call <vilib>:"Check if File or Folder Exists.vi"("error in (no error)"=w183, "path"=w180) -> ("error out"=w179:errorcluster, "file or folder exists?"=w176:bool, "dup path"=w177:path)  [unwired: 7 in]
              n70 = case shown="False" w176 {
                tunnel: w179 -> [w186 w187]
                tunnel: [w185 w187] -> w178
                tunnel: w177 -> [w184 _]
                frame False {
                  n71 = Create Folder(path (use dialog)=w184, error in=w186) -> (error out=w185:errorcluster)  [unwired: 1 in, 2 out]
                }
                frame True {
                }
              }
            }
          }
          frame "Update Folder Data" {
            # "Update folder data if user update the Username"
            n72 = call "FGV - Data Path.vi"("FGV State"=State_-_FGV."Read", "Error In"=w198) -> ("Error Out"=w189:errorcluster, "Path Out"=w197:path)  [unwired: 8 in]
            n73 = Unbundle By Name(w195) -> ("Old Username"=w194:string)
            n74 = local read "Username:"() -> (w192:string)
            n75 = Build Path(base path=w197, name or relative path="Data") -> (appended path=w193:path)
            n76 = Build Path(base path=w193, name or relative path=w194) -> (appended path=w191:path)
            n77 = Build Path(base path=w193, name or relative path=w192) -> (appended path=w190:path)
            n78 = Move(source path=w191, error in=w189, 10:w190) -> (error out=w188:errorcluster)  [unwired: 2 in, 2 out]
          }
          frame "Logout" {
            # "Logout required when user changed their username"
            n79 = Unbundle By Name(w212) -> ("Old Username"=w211:string)
            n80 = call "FGV - Login Status.vi"("Action"=enum16{"Read", "Write"}."Read", "Error In"=w209) -> ("Error Out"=w207:errorcluster, "Username Out"=w208:string)  [unwired: 7 in, 1 out]
            n81 = Equal?(x=w211, y=w208) -> (x = y?=w206:bool)
            n82 = case shown="True" w206 {
              tunnel: [w216 w219] -> w205
              tunnel: w207 -> [w216 w221]
              frame False {
                # "Other username changed. Ignore"
              }
              frame True {
                # "Own username changed. Logout"
                n83 = call "Gen - Popup Single Button (Auto Close).vi"("Type"=enum16{"Error", "Info"}."Info", "Error in"=w221, "Message in"="You have changed your username. Logout is required.\n\nPlease login again to continue.", "Header"="Logout") -> ("Error out"=w220:errorcluster)  [unwired: 6 in, 1 out]
                n84 = call "eFGV - Logout.vi"("Action"=State_-_eFGV."Write", "Error In"=w220, "Logout In"=TRUE) -> ("Error Out"=w219:errorcluster)  [unwired: 6 in, 2 out]
              }
            }
            n85 = property on="Tab Control" class="TabCtl (strict)"(error in=w205, "Value"=T1."Table" ("Tab Control")) -> (error out=w204:errorcluster)  [unwired: 1 in, 1 out]
          }
          frame "Idle", Default {
            n86 = event shown="[10] \"Back 1\", \"Back 2\", \"Back 3\": Value Change" {
              selector: w227 -> [_ _ _ _ _ _ _ _ _ _ _ _ _ _ _ _ _ _ _ _ _ _ _ _ _ _ _ _ _ _ _]
              dyn-events: [_ _ _ _ _ _ _ _ _ _ _ _ _ _ _ _ _ _ _ _ _ _ _ _ _ _ _ _ _ _ _] -> w228
              timeout: _ -> [_ _ _ _ _ _ _ _ _ _ _ _ _ _ _ _ _ _ _ _ _ _ _ _ _ _ _ _ _ _ _]
              tunnel: [State_-_Module_User_Management."Idle" State_-_Module_User_Management."Idle" State_-_Module_User_Management."Save User Authorization Info" State_-_Module_User_Management."Idle" State_-_Module_User_Management."Idle" State_-_Module_User_Management."Save User Authorization Info" State_-_Module_User_Management."Idle" State_-_Module_User_Management."Idle" State_-_Module_User_Management."Verify New User" State_-_Module_User_Management."Idle" State_-_Module_User_Management."Idle" State_-_Module_User_Management."Idle" State_-_Module_User_Management."Idle" w366 State_-_Module_User_Management."Idle" w378 w386 w396 State_-_Module_User_Management."Update Config User Access" State_-_Module_User_Management."Idle" w413 State_-_Module_User_Management."Idle" w427 State_-_Module_User_Management."Idle" State_-_Module_User_Management."Idle" State_-_Module_User_Management."Save User Authorization Info" State_-_Module_User_Management."Idle" State_-_Module_User_Management."Idle" w496 State_-_Module_User_Management."Exit" State_-_Module_User_Management."Exit"] -> w225
              tunnel: [w235 w241 w248 w264 w288 w310 w320 w329 w335 w339 w341 w346 w361 w370 w374 w384 w391 w400 w405 w410 w419 w424 w433 w435 w441 w445 w466 w472 w497 w537 w540] -> w231
              tunnel: w232 -> [w235 w239 w249 w262 w285 w311 w318 w330 w335 w339 w342 w347 w360 w370 w373 w384 w391 w401 w405 w409 w419 w423 w433 w436 w442 w446 w467 w473 w503 w537 w540]
              tunnel: [w234 w243 w259 w266 w290 w314 w323 w332 w334 w338 w344 w349 w363 w369 w377 w383 w390 w393 w404 w412 w418 w426 w432 w438 w443 w451 w470 w476 w500 w536 w539] -> w229
              tunnel: w230 -> [w234 w243 w259 w266 w290 w314 w323 w332 w334 w338 w344 w349 w363 w369 w377 w383 w390 w402 w404 w412 w418 w426 w432 w438 w443 w451 w470 w476 w513 w536 w539]
              event Timeout {
                n87 = event-data() -> ()  [unwired: 1 in, 3 out]
              }
              event User Event {
                # "Reset tab to Table when active page."
                n88 = event-data() -> ("VI Name"=w238:string)  [unwired: 1 in]
                n89 = control-ref of="This VI"() -> (w240:refnum<vi>)
                n90 = call "Gen - Check for Active Page.vi"("Error In"=w239, "VI Name in"=w238, "This VI"=w240) -> ("Error Out"=w236:errorcluster, "Active Page?"=w237:bool)  [unwired: 6 in, 1 out]
                n91 = case shown="True" w237 {
                  tunnel: [w244 w246] -> w241
                  tunnel: w236 -> [w244 w245]
                  frame False {
                  }
                  frame True {
                    n92 = property on="Tab Control" class="TabCtl (strict)"(error in=w245, "Value"=T1."Table" ("Tab Control")) -> (error out=w246:errorcluster)  [unwired: 1 in, 1 out]
                  }
                }
              }
              event "Filter:": Value Change {
                n93 = event-data() -> ("NewVal"=w250:string)  [unwired: 1 in]
                n94 = String Length(string=w250) -> (length=w254:i32)
                n95 = Multiply(x=w254, y=8 ("length")) -> (x*y=w255:i32)
                n96 = In Range and Coerce(upper limit=72, x=w255, lower limit=48) -> (coerced(x)=w256:i32)  [unwired: 1 out]
                n97 = To Unsigned Long Integer(number=w256) -> (unsigned 32bit integer=w257:u32)
                n98 = property on="Filter:" class="CmbBox"(error in=w249, "Width"=w257) -> (error out=w248:errorcluster)  [unwired: 1 in, 1 out]
              }
              event "Search Bar": Mouse Enter {
                n99 = event-data() -> ("CtlRef"=w263:refnum<vi>)  [unwired: 1 in, 3 out]
                n100 = property class="Str"(reference=w263, error in=w262) -> (error out=w261:errorcluster, "Key Focus"=w260:bool)  [unwired: 1 out]
                n101 = case shown="False" w260 {
                  tunnel: [w272 w283] -> w264
                  tunnel: w261 -> [w267 w283]
                  frame False {
                    n102 = property on="Search By:" class="RadioBtnsControl (strict)"(error in=w267) -> (error out=w269:errorcluster, "Value"=w271:T2)  [unwired: 1 in, 1 out]
                    n103 = case shown="\"L\", Default" w271 {
                      tunnel: [w280 w282] -> w270
                      tunnel: w269 -> [w280 w282]
                      tunnel: ["Search Name" "Search Username"] -> w268
                      frame "L", Default {
                      }
                      frame "R" {
                      }
                    }
                    n104 = property on="Search Bar" class="Str"(error in=w270) -> (error out=w277:errorcluster, "Value"=w273:string)  [unwired: 1 in, 1 out]
                    n105 = Equal?(x=w268, y=w273) -> (x = y?=w276:bool)
                    n106 = Select(t="", s=w276, f=w273) -> (s? t:f=w275:string)
                    n107 = property on="Search Bar" class="Str"(error in=w277, "Value"=w275, "Text.TextColor"=u32 0) -> (error out=w272:errorcluster)  [unwired: 1 in, 1 out]
                  }
                  frame True {
                  }
                }
              }
              event "Search Bar": Mouse Leave {
                n108 = event-data() -> ("CtlRef"=w287:refnum<vi>)  [unwired: 1 in, 3 out]
                n109 = property class="Str"(reference=w287, error in=w285) -> (error out=w286:errorcluster, "Key Focus"=w284:bool)  [unwired: 1 out]
                n110 = case shown="False" w284 {
                  tunnel: [w292 w308] -> w288
                  tunnel: w286 -> [w291 w308]
                  frame False {
                    n111 = property on="Search By:" class="RadioBtnsControl (strict)"(error in=w291) -> (error out=w302:errorcluster, "Value"=w303:T2)  [unwired: 1 in, 1 out]
                    n112 = case shown="\"L\", Default" w303 {
                      tunnel: [w305 w307] -> w294
                      tunnel: w302 -> [w305 w307]
                      tunnel: ["Search Name" "Search Username"] -> w293
                      frame "L", Default {
                      }
                      frame "R" {
                      }
                    }
                    n113 = property on="Search Bar" class="Str"(error in=w294) -> (error out=w297:errorcluster, "Value"=w299:string)  [unwired: 1 in, 1 out]
                    n114 = Empty String/Path?(string/path=w299) -> (empty?=w300:bool)
                    n115 = Select(t=w293, s=w300, f=w299) -> (s? t:f=w298:string)
                    n116 = Select(t=u32 7895160, s=w300, f=u32 0) -> (s? t:f=w301:u32)
                    n117 = property on="Search Bar" class="Str"(error in=w297, "Value"=w298, "Text.TextColor"=w301) -> (error out=w292:errorcluster)  [unwired: 1 in, 1 out]
                  }
                  frame True {
                  }
                }
              }
              event "Clear Search": Value Change {
                n118 = event-data() -> ()  [unwired: 1 in, 6 out]
                n119 = local write "Search Bar"("") -> ()
                n120 = property on="Clear Search" class="Bool"(error in=w311, "Visible"=FALSE) -> (error out=w310:errorcluster)  [unwired: 1 in, 1 out]
              }
              event Value Change {
                n121 = event-data() -> ("NewVal"=w319:T2)  [unwired: 1 in]
                n122 = case shown="\"L\", Default" w319 {
                  tunnel: ["Search Name" ("Search Bar") "Search Username" ("Search Bar")] -> w321
                  tunnel: w318 -> [w324 w326]
                  tunnel: [w324 w326] -> w317
                  frame "L", Default {
                  }
                  frame "R" {
                  }
                }
                n123 = property on="Search Bar" class="Str"(error in=w317, "Value"=w321, "Text.TextColor"=u32 7895160, "Key Focus"=FALSE) -> (error out=w320:errorcluster)  [unwired: 1 in, 1 out]
              }
              event "Cancel Create User": Value Change {
                n124 = event-data() -> ()  [unwired: 1 in, 6 out]
                n125 = property on="Tab Control" class="TabCtl (strict)"(error in=w330, "Value"=T1."Table" ("Tab Control")) -> (error out=w329:errorcluster)  [unwired: 1 in, 1 out]
              }
              event "Create User": Value Change {
                n126 = event-data() -> ()  [unwired: 1 in, 6 out]
              }
              event "User Information": Mouse Down {
                n127 = event-data() -> ()  [unwired: 1 in, 8 out]
                n128 = local write "Search User"("") -> ()
              }
              event "Back 1", "Back 2", "Back 3": Value Change {
                # "Back to List User Page"
                n129 = event-data() -> ()  [unwired: 1 in, 2 out]
                n130 = property on="Tab Control" class="TabCtl (strict)"(error in=w342, "Value"=T1."Table" ("Tab Control")) -> (error out=w341:errorcluster)  [unwired: 1 in, 1 out]
              }
              event "Config: Access Level": Value Change {
                n131 = event-data() -> ()  [unwired: 1 in, 1 out]
                n132 = property on="Config: Reset Page" class="Bool"(error in=w347, "DisabledEnum"=T14."Disabled and Grayed Out" ("Disabled")) -> (error out=w346:errorcluster)  [unwired: 1 in, 1 out]
              }
              event "Config: Accessible Page": Mouse Down? {
                n133 = event-data() -> ()  [unwired: 1 in, 1 out]
                n134 = property on="Config: Add Page" class="Bool"(error in=w360, "DisabledEnum"=T14."Disabled and Grayed Out" ("Disabled")) -> (error out=w355:errorcluster)  [unwired: 1 in, 1 out]
                n135 = property on="Config: Accessible Page" class="LstBox (strict)"(error in=w355) -> (error out=w354:errorcluster, "Item Names"=w358:string[])  [unwired: 1 in, 1 out]
                n136 = Array Size(array=w358) -> (size(s)=w357:i32)
                n137 = Equal?(x=w357, y=1) -> (x = y?=w350:bool)
                "Delete Msg" <- w350
                n138 = Select(t=T14."Disabled and Grayed Out", s=w350, f=T14."Enabled" ("Disabled")) -> (s? t:f=w351:T14)
                n139 = property on="Config: Delete Page" class="Bool"(error in=w354, "DisabledEnum"=w351) -> (error out=w361:errorcluster)  [unwired: 1 in, 1 out]
                n140 = event-data() -> ()  [unwired: 5 in, 1 out]
              }
              event "Config: Add Page": Value Change {
                n141 = event-data() -> ("Time"=w365:u32)  [unwired: 1 in]
                n142 = call "Gen - Check for Repeating User Event.vi"("Time"=w365) -> ("Repeat?"=w364:bool)  [unwired: 10 in]
                n143 = Select(t=State_-_Module_User_Management."Add User Access Page", s=w364, f=State_-_Module_User_Management."Idle") -> (s? t:f=w366:T9)
              }
              event "Config: All Page": Mouse Down? {
                n144 = event-data() -> ()  [unwired: 1 in, 1 out]
                n145 = property on="Config: Add Page" class="Bool"(error in=w373, "DisabledEnum"=T14."Enabled" ("Disabled")) -> (error out=w375:errorcluster)  [unwired: 1 in, 1 out]
                n146 = property on="Config: Delete Page" class="Bool"(error in=w375, "DisabledEnum"=T14."Disabled and Grayed Out" ("Disabled")) -> (error out=w374:errorcluster)  [unwired: 1 in, 1 out]
                n147 = event-data() -> ()  [unwired: 5 in, 1 out]
              }
              event "Config: Delete Page": Value Change {
                n148 = event-data() -> ("Time"=w382:u32)  [unwired: 1 in]
                n149 = call "Gen - Check for Repeating User Event.vi"("Time"=w382) -> ("Repeat?"=w380:bool)  [unwired: 10 in]
                n150 = Select(t=State_-_Module_User_Management."Reset User Access Page", s=w380, f=State_-_Module_User_Management."Idle") -> (s? t:f=w378:T9)
              }
              event "Config: Reset Page": Value Change {
                n151 = event-data() -> ("Time"=w389:u32)  [unwired: 1 in]
                n152 = call "Gen - Check for Repeating User Event.vi"("Time"=w389) -> ("Repeat?"=w388:bool)  [unwired: 10 in]
                n153 = Select(t=State_-_Module_User_Management."Reset User Access Page", s=w388, f=State_-_Module_User_Management."Idle") -> (s? t:f=w386:T9)
              }
              event "Config: Update": Value Change {
                n154 = event-data() -> ("Time"=w394:u32)  [unwired: 1 in]
                n155 = property on="Config: Reset Page" class="Bool"(error in=w401, "DisabledEnum"=T14."Enabled" ("Disabled")) -> (error out=w400:errorcluster)  [unwired: 1 in, 1 out]
                n156 = Bundle By Name(cluster=w402, "Update User"=TRUE) -> (w393:T8)
                n157 = call "Gen - Check for Repeating User Event.vi"("Time"=w394) -> ("Repeat?"=w398:bool)  [unwired: 10 in]
                n158 = Select(t=State_-_Module_User_Management."Edit User Info", s=w398, f=State_-_Module_User_Management."Idle") -> (s? t:f=w396:T9)
              }
              event "Manage: Access Level": Value Change {
                n159 = event-data() -> ()  [unwired: 1 in, 6 out]
              }
              event "Manage: Accessible Page": Mouse Down? {
                n160 = event-data() -> ()  [unwired: 1 in, 1 out]
                n161 = property on="Manage: Add Page" class="Bool"(error in=w409, "DisabledEnum"=T14."Disabled and Grayed Out" ("Disabled")) -> (error out=w408:errorcluster)  [unwired: 1 in, 1 out]
                n162 = property on="Manage: Delete Page" class="Bool"(error in=w408, "DisabledEnum"=T14."Enabled" ("Disabled")) -> (error out=w410:errorcluster)  [unwired: 1 in, 1 out]
                n163 = event-data() -> ()  [unwired: 5 in, 1 out]
              }
              event "Manage: Add Page": Value Change {
                n164 = event-data() -> ("Time"=w417:u32)  [unwired: 1 in]
                n165 = call "Gen - Check for Repeating User Event.vi"("Time"=w417) -> ("Repeat?"=w416:bool)  [unwired: 10 in]
                n166 = Select(t=State_-_Module_User_Management."Add Config Access Page", s=w416, f=State_-_Module_User_Management."Idle") -> (s? t:f=w413:T9)
              }
              event "Manage: All Page": Mouse Down? {
                n167 = event-data() -> ()  [unwired: 1 in, 1 out]
                n168 = property on="Manage: Add Page" class="Bool"(error in=w423, "DisabledEnum"=T14."Enabled" ("Disabled")) -> (error out=w422:errorcluster)  [unwired: 1 in, 1 out]
                n169 = property on="Manage: Delete Page" class="Bool"(error in=w422, "DisabledEnum"=T14."Disabled and Grayed Out" ("Disabled")) -> (error out=w424:errorcluster)  [unwired: 1 in, 1 out]
                n170 = event-data() -> ()  [unwired: 5 in, 1 out]
              }
              event "Manage: Delete Page": Value Change {
                n171 = event-data() -> ("Time"=w431:u32)  [unwired: 1 in]
                n172 = call "Gen - Check for Repeating User Event.vi"("Time"=w431) -> ("Repeat?"=w430:bool)  [unwired: 10 in]
                n173 = Select(t=State_-_Module_User_Management."Remove Config Access Page", s=w430, f=State_-_Module_User_Management."Idle") -> (s? t:f=w427:T9)
              }
              event "Setting": Value Change {
                n174 = event-data() -> ()  [unwired: 1 in, 6 out]
                n175 = property on="Tab Control" class="TabCtl (strict)"(error in=w436, "Value"=T1."Config" ("Tab Control")) -> (error out=w435:errorcluster)  [unwired: 1 in, 1 out]
              }
              event "Add User": Value Change {
                w439 = ""
                n176 = event-data() -> ()  [unwired: 1 in, 1 out]
                n177 = local write "New Name:"(w439) -> ()
                n178 = local write "New Username:"(w439) -> ()
                n179 = local write "New Password:"(w439) -> ()
                n180 = local write "Re-Type Password:"(w439) -> ()
                n181 = local write "New Access Level:"(w439) -> ()
                n182 = property on="Tab Control" class="TabCtl (strict)"(error in=w442, "Value"=T1."New User" ("Tab Control")) -> (error out=w441:errorcluster)  [unwired: 1 in, 1 out]
              }
              event "Search Bar": Value Change {
                n183 = event-data() -> ("NewVal"=w448:string)  [unwired: 1 in]
                n184 = Empty String/Path?(string/path=w448) -> (empty?=w449:bool)
                n185 = Not(x=w449) -> (.not. x?=w447:bool)
                n186 = property on="Clear Search" class="Bool"(error in=w446, "Visible"=w447) -> (error out=w445:errorcluster)  [unwired: 1 in, 1 out]
              }
              event "User Information": Mouse Up {
                n187 = event-data() -> ("CtlRef"=w468:refnum<vi>)  [unwired: 1 in]
                n188 = property class="Arr"(reference=w468, error in=w467) -> (reference out=w465:refnum<vi>, error out=w463:errorcluster, "Value"=w464:variant, "Number of Rows"=w458:u32, "Index Values"=w455:u32[])
                n189 = local read "User Information"() -> (w461:T3[])
                n190 = Variant To Data(error in=w463, type=w461, Variant=w464) -> (data=w460:T3[], error out=w462:errorcluster)
                n191 = Array Size(array=w460) -> (size(s)=w459:i32)
                n192 = To Unsigned Long Integer(number=w459) -> (unsigned 32bit integer=w452:u32)
                n193 = Subtract(x=w452, y=w458) -> (x-y=w457:u32)
                n194 = Build Array(w457) -> (w454:u32[])
                n195 = Less?(x=w454, y=w455) -> (x < y?=w456:bool)
                n196 = Select(t=w454, s=w456, f=w455) -> (s? t:f=w453:u32[])
                n197 = property class="Arr"(reference=w465, error in=w462, "Index Values"=w453) -> (error out=w466:errorcluster)  [unwired: 1 out]
              }
              event "User Information": Mouse Wheel {
                n198 = event-data() -> ("Delta"=w471:i32, "CtlRef"=w474:refnum<vi>)  [unwired: 1 in]
                n199 = case shown="0, Default" w471 {
                  tunnel: w474 -> [w489 _ _]
                  tunnel: w473 -> [w488 w490 w491]
                  tunnel: [w486 w490 w491] -> w472
                  frame -1 {
                    # "Down"
                    n200 = property class="Arr"(reference=w489, error in=w488) -> (reference out=w487:refnum<vi>, error out=w484:errorcluster, "Value"=w485:variant, "Number of Rows"=w479:u32)
                    n201 = local read "User Information"() -> (w482:T3[])
                    n202 = Variant To Data(error in=w484, type=w482, Variant=w485) -> (data=w481:T3[], error out=w483:errorcluster)
                    n203 = Array Size(array=w481) -> (size(s)=w480:i32)
                    n204 = Subtract(x=w480, y=w479) -> (x-y=w478:u32)
                    n205 = Build Array(w478) -> (w477:u32[])
                    n206 = property class="Arr"(reference=w487, error in=w483, "Index Values"=w477) -> (error out=w486:errorcluster)  [unwired: 1 out]
                  }
                  frame 0, Default {
                  }
                  frame 1 {
                    # "Up"
                  }
                }
              }
              event "User Information": Value Change {
                # "Check clicked control. Next case depending on index (clicked control)"
                n207 = event-data() -> ("OldVal"=w495:T3[], "NewVal"=w507:T3[])  [unwired: 1 in, 1 out]
                n208 = for {
                  tunnel: w507 -> [w534] mode=indexing
                  tunnel: w495 -> [w533] mode=indexing
                  tunnel: [w532] -> w510 mode=indexing
                  tunnel: [w531] -> w501
                  tunnel: w503 -> [w531]
                  tunnel: [w530] -> w499
                  i -> [w530]
                  stop <- w532 stop-if-true
                  n209 = Not Equal?(x=w533, y=w534) -> (x != y?=w532:bool)
                }
                n210 = Bundle By Name(cluster=w513, "Selected Row"=w499) -> (w500:T8)
                n211 = Search 1D Array(1D array=w510, element=TRUE) -> (index of element=w511:i32)  [unwired: 1 in]
                n212 = Index Array(array=w507, index=w511) -> (element=w509:T3)
                n213 = Index Array(array=w495, index=w511) -> (element=w508:T3)
                n214 = Not Equal?(x=w509, y=w508) -> (x != y?=w506:T23)
                n215 = Cluster To Array(cluster=w506) -> (array=w505:bool[])
                n216 = To Variant(anything=w495) -> (Variant=w494:variant)
                n217 = Search 1D Array(1D array=w505, element=TRUE) -> (index of element=w502:i32)  [unwired: 1 in]
                n218 = case shown="7" w502 {
                  tunnel: [w516 w519 w524 w526] -> w498
                  tunnel: w501 -> [w516 w520 w524 w528]
                  tunnel: [State_-_Module_User_Management."Idle" State_-_Module_User_Management."Update Selected User" State_-_Module_User_Management."Block" State_-_Module_User_Management."Check Logged User"] -> w496
                  tunnel: w494 -> [_ w518 _ w527]
                  tunnel: [T1."Table" ("Tab Control") T1."Edit User" ("Tab Control") T1."Table" ("Tab Control") T1."Table" ("Tab Control")] -> w492
                  frame 0, Default {
                  }
                  frame 5 {
                    # "Edit"
                    n219 = property on="User Information" class="Arr"(error in=w520, "Value"=w518) -> (error out=w519:errorcluster)  [unwired: 1 in, 1 out]
                  }
                  frame 6 {
                    # "Block"
                  }
                  frame 7 {
                    # "Remove"
                    n220 = property on="User Information" class="Arr"(error in=w528, "Value"=w527) -> (error out=w526:errorcluster)  [unwired: 1 in, 1 out]
                  }
                }
                n221 = local write "Search User"("") -> ()
                n222 = property on="Tab Control" class="TabCtl (strict)"(error in=w498, "Value"=w492) -> (error out=w497:errorcluster)  [unwired: 1 in, 1 out]
              }
              event User Event {
                n223 = event-data() -> ()  [unwired: 1 in, 4 out]
              }
              event "Stop": Value Change {
                n224 = event-data() -> ()  [unwired: 1 in, 6 out]
              }
            }
          }
          frame "Reset User Access Page" {
            n225 = Unbundle By Name(w572) -> ("Selected Row"=w556:i32)
            n226 = property on="User Information T" class="MCListbox (strict)"(error in=w568) -> (error out=w567:errorcluster, "ItemNames"=w571:string[][])  [unwired: 1 in, 1 out]
            n227 = To Long Integer(number=Header_-_User_Management."Access Level" ("Header - User Management")) -> (32bit integer=w570:i32)
            n228 = Index Array(array=w571, index (row)=w556, index (col)=w570) -> (element=w565:string)
            n229 = property on="Config: Access Level" class="CmbBox"(error in=w567) -> (error out=w564:errorcluster, "Strings[]"=w566:string[])  [unwired: 1 in, 1 out]
            n230 = Search 1D Array(1D array=w566, element=w565) -> (index of element=w553:i32)  [unwired: 1 in]
            n231 = property on="Access Page T" class="LstBox (strict)"(error in=w564) -> (error out=w545:errorcluster, "Item Names"=w552:string[])  [unwired: 1 in, 1 out]
            n232 = call "Gen - System Config.vi"() -> ("Data Out"=w546:T18)  [unwired: 11 in]
            n233 = Index Array(array=w552, index=w553) -> (element=w549:string)
            n234 = Unbundle By Name(w546) -> ("Button.Text"=w547:string[], "Page Module"=w548:string[])
            n235 = call <vilib>:"Delimited String to 1D String Array.vi"("delimiter"=",", "delimited string"=w549) -> ("string array"=w551:string[])  [unwired: 9 in]
            n236 = Sort 1D Array(array=w551) -> (sorted array=w554:string[])
            n237 = call "Gen - Remove Empty String Array.vi"("Data Array"=w554) -> ("Data Out"=w543:string[])  [unwired: 10 in]
            n238 = call "User - Filter List.vi"("Error In"=w545, "Data to Search"=w543, "Search From"=w548, "All List"=w547) -> ("Error Out"=w544:errorcluster, "Data Out"=w542:string[])  [unwired: 6 in]
            n239 = call "Gen - Remove Empty String Array.vi"("Data Array"=w542) -> ("Data Out"=w541:string[])  [unwired: 10 in]
            n240 = property on="Config: Accessible Page" class="LstBox (strict)"(error in=w544, "Item Names"=w541) -> (error out=w563:errorcluster)  [unwired: 1 in, 1 out]
            n241 = call <vilib>:"1D String Array to Delimited String.vi"("delimiter"=",", "string array"=w543) -> ()  [unwired: 9 in, 1 out]
            n242 = property on="User Information T" class="MCListbox (strict)"(error in=w563) -> (error out=w559:errorcluster, "ItemNames"=w562:string[][])  [unwired: 1 in, 1 out]
            n243 = To Long Integer(number=Header_-_User_Management."Access Page" ("Header - User Management")) -> (32bit integer=w561:i32)
            n244 = Replace Array Subset(array=w562, new element=w549, index (row)=w556, index (col)=w561) -> (w560:string[][])
            n245 = property on="User Information T" class="MCListbox (strict)"(error in=w559, "ItemNames"=w560) -> (error out=w555:errorcluster)  [unwired: 1 in, 1 out]
          }
          frame "Add User Access Page" {
            n246 = property on="Config: All Page" class="LstBox (strict)"(error in=w601) -> (error out=w598:errorcluster, "Item Names"=w600:string[], "Value"=w599:i32)  [unwired: 1 in, 1 out]
            n247 = Index Array(array=w600, index=w599) -> (element=w596:string)
            n248 = property on="Config: Accessible Page" class="LstBox (strict)"(error in=w598) -> (error out=w595:errorcluster, "Item Names"=w597:string[])  [unwired: 1 in, 1 out]
            n249 = Insert Into Array(array=w597, new element=w596) -> (w594:string[])  [unwired: 1 in]
            n250 = call "Remove Duplicates From 1D Array.vim"("array"=w594) -> ("array with duplicates removed"=w589:string[])  [unwired: 10 in]
            n251 = Sort 1D Array(array=w589) -> (sorted array=w577:string[])
            n252 = call "Gen - System Config.vi"() -> ("Data Out"=w583:T18)  [unwired: 11 in]
            n253 = call "Gen - Remove Empty String Array.vi"("Data Array"=w577) -> ("Data Out"=w576:string[])  [unwired: 10 in]
            n254 = Unbundle By Name(w583) -> ("Page Module"=w581:string[], "Button.Text"=w582:string[])
            n255 = property on="Config: Accessible Page" class="LstBox (strict)"(error in=w595, "Item Names"=w576) -> (error out=w580:errorcluster)  [unwired: 1 in, 1 out]
            n256 = call "User - Filter List.vi"("Error In"=w580, "Data to Search"=w576, "Search From"=w582, "All List"=w581) -> ("Error Out"=w579:errorcluster, "Data Out"=w578:string[])  [unwired: 6 in]
            n257 = call <vilib>:"1D String Array to Delimited String.vi"("delimiter"=",", "string array"=w578) -> ("delimited string"=w587:string)  [unwired: 9 in]
            n258 = property on="User Information T" class="MCListbox (strict)"(error in=w579) -> (error out=w585:errorcluster, "ItemNames"=w593:string[][])  [unwired: 1 in, 1 out]
            n259 = Unbundle By Name(w602) -> ("Selected Row"=w592:i32)
            n260 = To Long Integer(number=Header_-_User_Management."Access Page" ("Header - User Management")) -> (32bit integer=w590:i32)
            n261 = Replace Array Subset(array=w593, new element=w587, index (row)=w592, index (col)=w590) -> (w586:string[][])
            n262 = property on="User Information T" class="MCListbox (strict)"(error in=w585, "ItemNames"=w586) -> (error out=w584:errorcluster)  [unwired: 1 in, 1 out]
          }
          frame "Remove User Access Page" {
            n263 = property on="Config: Accessible Page" class="LstBox (strict)"(error in=w608) -> (error out=w624:errorcluster, "Item Names"=w626:string[], "Value"=w625:i32)  [unwired: 1 in, 1 out]
            n264 = Delete From Array(array=w626, index=w625) -> (array with subset deleted=w607:string[])  [unwired: 1 in, 1 out]
            n265 = call "Gen - Remove Empty String Array.vi"("Data Array"=w607) -> ("Data Out"=w606:string[])  [unwired: 10 in]
            n266 = call "Gen - System Config.vi"() -> ("Data Out"=w614:T18)  [unwired: 11 in]
            n267 = Unbundle By Name(w614) -> ("Page Module"=w612:string[], "Button.Text"=w613:string[])
            n268 = property on="Config: Accessible Page" class="LstBox (strict)"(error in=w624, "Item Names"=w606) -> (error out=w611:errorcluster)  [unwired: 1 in, 1 out]
            n269 = call "User - Filter List.vi"("Error In"=w611, "Data to Search"=w606, "Search From"=w613, "All List"=w612) -> ("Error Out"=w609:errorcluster, "Data Out"=w610:string[])  [unwired: 6 in]
            n270 = call <vilib>:"1D String Array to Delimited String.vi"("delimiter"=",", "string array"=w610) -> ("delimited string"=w618:string)  [unwired: 9 in]
            n271 = Unbundle By Name(w627) -> ("Selected Row"=w622:i32)
            n272 = property on="User Information T" class="MCListbox (strict)"(error in=w609) -> (error out=w617:errorcluster, "ItemNames"=w623:string[][])  [unwired: 1 in, 1 out]
            n273 = To Long Integer(number=Header_-_User_Management."Access Page" ("Header - User Management")) -> (32bit integer=w620:i32)
            n274 = Replace Array Subset(array=w623, new element=w618, index (row)=w622, index (col)=w620) -> (w615:string[][])
            n275 = property on="User Information T" class="MCListbox (strict)"(error in=w617, "ItemNames"=w615) -> (error out=w616:errorcluster)  [unwired: 1 in, 1 out]
          }
          frame "Save User Authorization Info" {
            n276 = property on="User Information T" class="MCListbox (strict)"(error in=w641, "Value"=-1 ("Multicolumn Listbox")) -> (error out=w640:errorcluster)  [unwired: 1 in, 1 out]
            n277 = Unbundle By Name(w638) -> ("Path User Info"=w645:path)
            n278 = property on="User Information T" class="MCListbox (strict)"(error in=w640) -> (error out=w632:errorcluster, "ItemNames"=w633:string[][])  [unwired: 1 in, 1 out]
            n279 = call "FGV - Authorization Data.vi"("State - FGV"=State_-_FGV."Write", "Error In"=w632, "Data In"=w633) -> ("Error Out"=w631:errorcluster)  [unwired: 7 in, 1 out]
            n280 = To Variant(anything=w633) -> (Variant=w637:variant)
            n281 = call "aFGV - Binary File.vi"("State"=enum16{"Read", "Write"}."Write", "Error In"=w631, "Path"=w645, "Data in"=w637) -> ("Error Out"=w635:errorcluster)  [unwired: 6 in, 1 out]
          }
          frame "Search User" {
            # "Search define user."
            n282 = property on="Search By:" class="RadioBtnsControl (strict)"(error in=w664) -> (error out=w661:errorcluster, "Value"=w660:T2)  [unwired: 1 in, 1 out]
            n283 = Equal To 0?(x=w660) -> (x = 0?=w647:bool)
            n284 = property on="Search Bar" class="Str"(error in=w661) -> (error out=w659:errorcluster, "Value"=w653:string)  [unwired: 1 in, 1 out]
            n285 = Unbundle By Name(w662) -> ("User Information.Filtered"=w654:T3[])
            n286 = Empty String/Path?(string/path=w653) -> (empty?=w656:bool)
            n287 = Equal?(x=w653, y="Search Name") -> (x = y?=w649:bool)
            n288 = Equal?(x=w653, y="Search Username") -> (x = y?=w648:bool)
            n289 = for {
              tunnel: w653 -> [w679]
              tunnel: [w674] -> w658
              tunnel: w659 -> [w674]
              tunnel: w654 -> [w670] mode=indexing
              tunnel: [w670] -> w646 mode=indexing if=w673
              tunnel: w647 -> [w672]
              n290 = Unbundle By Name(w670) -> ("Name"=w671:string, "Username"=w668:string)
              n291 = Select(t=w671, s=w672, f=w668) -> (s? t:f=w669:string)
              n292 = To Lower Case(string=w669) -> (all lower case string=w676:string)
              n293 = To Lower Case(string=w679) -> (all lower case string=w675:string)
              n294 = Match Pattern(string=w676, regular expression=w675) -> (match substring=w678:string)  [unwired: 1 in, 3 out]
              n295 = Empty String/Path?(string/path=w678) -> (empty?=w677:bool)
              n296 = Not(x=w677) -> (.not. x?=w673:bool)
            }
            n297 = Compound Arithmetic op=AND(w656, w649, w648) -> (w650:bool)
            n298 = Select(t=w654, s=w650, f=w646) -> (s? t:f=w655:T3[])
            n299 = To Variant(anything=w655) -> (Variant=w657:variant)
            n300 = property on="User Information" class="Arr"(error in=w658, "Value"=w657) -> (error out=w663:errorcluster)  [unwired: 1 in, 1 out]
          }
          frame "Verify New User" {
            # "Used username"
            # "Verify all information for new user. Check either username is unique and password is match."
            n301 = property on="User Info T" class="MCListbox (strict)"(error in=w711) -> (error out=w684:errorcluster, "ItemNames"=w705:string[][])  [unwired: 1 in, 1 out]
            n302 = local read "New Username:"() -> (w703:string)
            n303 = To Long Integer(number=Header_-_User_Management."Username" ("Header - User Management")) -> (32bit integer=w710:i32)
            n304 = Index Array(array=w705, index (col)=w710) -> (element=w709:string[])  [unwired: 1 in]
            n305 = call <vilib>:"Space Constant.vi"() -> ("String"=w707:string)
            n306 = Match Pattern(string=w703, regular expression=w707) -> (match substring=w706:string)  [unwired: 1 in, 3 out]
            n307 = Search 1D Array(1D array=w709, element=w703) -> (index of element=w708:i32)  [unwired: 1 in]
            n308 = Empty String/Path?(string/path="Staff Id") -> (empty?=w682:bool)
            n309 = Equal?(x="Re-Type Password:", y="New Password:") -> (x = y?=w693:bool)
            n310 = Empty String/Path?(string/path="New Name:") -> (empty?=w697:bool)
            n311 = Empty String/Path?(string/path="New Username:") -> (empty?=w696:bool)
            n312 = Empty String/Path?(string/path="New Password:") -> (empty?=w695:bool)
            n313 = Empty String/Path?(string/path="New Access Level:") -> (empty?=w694:bool)
            n314 = Not(x=w682) -> (.not. x?=w680:bool)
            n315 = Not(x=w697) -> (.not. x?=w692:bool)
            n316 = Not(x=w696) -> (.not. x?=w691:bool)
            n317 = Not(x=w695) -> (.not. x?=w690:bool)
            n318 = Not(x=w694) -> (.not. x?=w689:bool)
            n319 = Less Than 0?(x=w708) -> (x < 0?=w688:bool)
            n320 = Empty String/Path?(string/path=w706) -> (empty?=w687:bool)
            n321 = Compound Arithmetic op=AND(w693, w692, w691, w690, w689, w688, w687, w680) -> (w686:bool)
            n322 = case shown="True" w686 {
              tunnel: [w718 w723] -> w685
              tunnel: w684 -> [w717 w723]
              tunnel: [State_-_Module_User_Management."Idle" State_-_Module_User_Management."Create New User"] -> w683
              frame False {
                w715 = ""
                n323 = call "Gen - Popup Single Button (Auto Close).vi"("Type"=enum16{"Error", "Info"}."Error", "Error in"=w717, "Message in"="Error creating new user.\n\nPlease fill up all information and use unique username. ", "Header"="Create User") -> ("Error out"=w718:errorcluster)  [unwired: 6 in, 1 out]
                n324 = local write "New Name:"(w715) -> ()
                n325 = local write "New Username:"(w715) -> ()
                n326 = local write "New Password:"(w715) -> ()
                n327 = local write "Re-Type Password:"(w715) -> ()
                n328 = local write "New Access Level:"(w715) -> ()
                n329 = local write "Staff Id"(w715) -> ()
              }
              frame True {
              }
            }
          }
          frame "Create New User" {
            (unwired) TRUE
            # "Create new user and then update table"
            n330 = property on="User Info T" class="MCListbox (strict)"(error in=w748) -> (error out=w745:errorcluster, "ItemNames"=w747:string[][])  [unwired: 1 in, 1 out]
            n331 = property on="New Access Level:" class="CmbBox"(error in=w745) -> (error out=w744:errorcluster, "Strings[]"=w743:string[], "Value"=w742:string)  [unwired: 1 in, 1 out]
            n332 = Search 1D Array(1D array=w743, element=w742) -> (index of element=w740:i32)  [unwired: 1 in]
            n333 = local read "New Access Level:"() -> (w733:string)
            n334 = local read "New Username:"() -> (w735:string)
            n335 = local read "Staff Id"() -> (w724:string)
            n336 = local read "New Password:"() -> (w734:string)
            n337 = local read "New Name:"() -> (w736:string)
            n338 = property on="Access Page T" class="LstBox (strict)"(error in=w744) -> (error out=w746:errorcluster, "Item Names"=w741:string[])  [unwired: 1 in, 1 out]
            n339 = Index Array(array=w741, index=w740) -> (element=w738:string)
            n340 = Build Array(w736, w724, w735, w734, w733, "Unblock" ("element"), w738) -> (w737:string[])
            n341 = Insert Into Array(array=w747, new element=w737) -> (w729:string[][])  [unwired: 2 in]
            n342 = property on="User Information T" class="MCListbox (strict)"(error in=w746, "ItemNames"=w729) -> (error out=w731:errorcluster)  [unwired: 1 in, 1 out]
            n343 = control-ref of="User Information"() -> (w730:refnum<vi>)
            n344 = call "User - Update User Table.vi"("Error In"=w731, "Max visible row"=7, "User Infor Ref"=w730, "User Information"=w729) -> ("Error Out"=w728:errorcluster)  [unwired: 6 in, 1 out]
            n345 = disable-structure shown="Enabled" {
              disable-tunnel: w729 -> [w754 _]
              disable-tunnel: w728 -> [w753 w758]
              disable-tunnel: [w752 w758] -> w727
              frame Disabled {
                n346 = To Long Integer(number=Header_-_User_Management."Name" ("Header - User Management")) -> (32bit integer=w756:i32)
                n347 = Index Array(array=w754, index (col)=w756) -> (element=w757:string[])  [unwired: 1 in]
                n348 = property on="Search User" class="CmbBox"(error in=w753, "Strings[]"=w757) -> (error out=w752:errorcluster)  [unwired: 1 in, 1 out]
              }
              frame Enabled {
              }
            }
            n349 = flat-sequence {
              tunnel: w727 -> [w761]
              tunnel: [w760] -> w726
              frame #0 {
                n350 = property on="Tab Control" class="TabCtl (strict)"(error in=w761, "Value"=T15."Table" ("Tab Control")) -> (error out=w760:errorcluster)  [unwired: 1 in, 1 out]
              }
            }
          }
          frame "Update Authrorization Data" {
            n351 = property on="User Information T" class="MCListbox (strict)"(error in=w762) -> (error out=w763:errorcluster, "ItemNames"=w764:string[][])  [unwired: 1 in, 1 out]
            n352 = call "FGV - Authorization Data.vi"("State - FGV"=State_-_FGV."Write", "Error In"=w763, "Data In"=w764) -> ("Error Out"=w766:errorcluster)  [unwired: 7 in, 1 out]
          }
          frame "Update Selected User" {
            # "Update info for selected user."
            n353 = Unbundle By Name(w800) -> ("Selected Row"=w798:i32)  [unwired: 1 out]
            n354 = property on="User Information T" class="MCListbox (strict)"(error in=w801) -> (error out=w776:errorcluster, "ItemNames"=w799:string[][])  [unwired: 1 in, 1 out]
            n355 = Index Array(array=w799, index (row)=w798) -> (element=w796:string[])  [unwired: 1 in]
            n356 = To Long Integer(number=Header_-_User_Management."Name" ("Header - User Management")) -> (32bit integer=w795:i32)
            n357 = To Long Integer(number=Header_-_User_Management."Username" ("Header - User Management")) -> (32bit integer=w789:i32)
            n358 = To Long Integer(number=Header_-_User_Management."Password" ("Header - User Management")) -> (32bit integer=w791:i32)
            n359 = To Long Integer(number=Header_-_User_Management."Access Level" ("Header - User Management")) -> (32bit integer=w790:i32)
            n360 = To Long Integer(number=Header_-_User_Management."Access Page" ("Header - User Management")) -> (32bit integer=w784:i32)
            n361 = Index Array(array=w796, index #1=w795, index #2=w789, index #3=w791, index #4=w790, index #5=w784) -> (element #1=w788:string, element #2=w773:string, element #3=w787:string, element #4=w786:string, element #5=w783:string)
            n362 = local write "Config: Access Level"(w786) -> ()
            n363 = call <vilib>:"Delimited String to 1D String Array.vi"("delimiter"=",", "delimited string"=w783) -> ("string array"=w777:string[])  [unwired: 9 in]
            n364 = local write "Name:"(w788) -> ()
            n365 = local write "Username:"(w773) -> ()
            n366 = local write "Password:"(w787) -> ()
            n367 = Bundle By Name(cluster=w800, "Old Username"=w773) -> (w774:T8)
            n368 = call "Gen - System Config.vi"() -> ("Data Out"=w780:T18)  [unwired: 11 in]
            n369 = Unbundle By Name(w780) -> ("Button.Text"=w778:string[], "Page Module"=w779:string[])
            n370 = call "User - Filter List.vi"("Error In"=w776, "Data to Search"=w777, "Search From"=w779, "All List"=w778) -> ("Error Out"=w775:errorcluster, "Data Out"=w772:string[])  [unwired: 6 in]
            n371 = call "Gen - Remove Empty String Array.vi"("Data Array"=w772) -> ("Data Out"=w771:string[])  [unwired: 10 in]
            n372 = property on="Config: Accessible Page" class="LstBox (strict)"(error in=w775, "Item Names"=w771) -> (error out=w781:errorcluster)  [unwired: 1 in, 1 out]
          }
          frame "Edit User Info" {
            # "Update info of selected user."
            n373 = Unbundle By Name(w811) -> ("Selected Row"=w822:i32)
            n374 = property on="User Information T" class="MCListbox (strict)"(error in=w839) -> (error out=w826:errorcluster, "ItemNames"=w812:string[][])  [unwired: 1 in, 1 out]
            n375 = Index Array(array=w812, index (row)=w822) -> (element=w838:string[])  [unwired: 1 in]
            n376 = call "Gen - System Config.vi"() -> ("Data Out"=w817:T18)  [unwired: 11 in]
            n377 = Unbundle By Name(w817) -> ("Page Module"=w819:string[], "Button.Text"=w818:string[])
            n378 = property on="Config: Accessible Page" class="LstBox (strict)"(error in=w826) -> (error out=w814:errorcluster, "Item Names"=w816:string[])  [unwired: 1 in, 1 out]
            n379 = local read "Config: Access Level"() -> (w827:string)
            n380 = call "User - Filter List.vi"("Error In"=w814, "Data to Search"=w816, "Search From"=w818, "All List"=w819) -> ("Error Out"=w813:errorcluster, "Data Out"=w815:string[])  [unwired: 6 in]
            n381 = Unbundle By Name(w811) -> ("Old Username"=w810:string)
            n382 = To Long Integer(number=Header_-_User_Management."Name" ("Header - User Management")) -> (32bit integer=w832:i32)
            n383 = To Long Integer(number=Header_-_User_Management."Username" ("Header - User Management")) -> (32bit integer=w831:i32)
            n384 = To Long Integer(number=Header_-_User_Management."Password" ("Header - User Management")) -> (32bit integer=w830:i32)
            n385 = To Long Integer(number=Header_-_User_Management."Access Level" ("Header - User Management")) -> (32bit integer=w829:i32)
            n386 = To Long Integer(number=Header_-_User_Management."Access Page" ("Header - User Management")) -> (32bit integer=w828:i32)
            n387 = call <vilib>:"1D String Array to Delimited String.vi"("delimiter"=",", "string array"=w815) -> ("delimited string"=w825:string)  [unwired: 9 in]
            n388 = Not Equal?(x=w810, y="Username:") -> (x != y?=w808:bool)
            n389 = Replace Array Subset(array=w838, new element #1="Name:", index #1=w832, new element #2="Username:", index #2=w831, new element #3="Password:", index #3=w830, new element #4=w827, index #4=w829, new element #5=w825, index #5=w828) -> (w821:string[])
            n390 = Bundle By Name(cluster=w811, "Username Updated?"=w808) -> (w809:T8)
            n391 = Replace Array Subset(array=w812, new element=w821, index (row)=w822) -> (w820:string[][])  [unwired: 1 in]
            n392 = property on="User Information T" class="MCListbox (strict)"(error in=w813, "ItemNames"=w820) -> (error out=w823:errorcluster)  [unwired: 1 in, 1 out]
          }
          frame "Check Logged User" {
            # "Check logged user. Prevent user to delete their account."
            n393 = Unbundle By Name(w857) -> ("Selected Row"=w854:i32)
            n394 = property on="User Information T" class="MCListbox (strict)"(error in=w856) -> (error out=w848:errorcluster, "ItemNames"=w855:string[][])  [unwired: 1 in, 1 out]
            n395 = Index Array(array=w855, index (row)=w854) -> (element=w852:string[])  [unwired: 1 in]
            n396 = To Long Integer(number=Header_-_User_Management."Username" ("Header - User Management")) -> (32bit integer=w851:i32)
            n397 = call "FGV - Login Status.vi"("Action"=enum16{"Read", "Write"}."Read", "Error In"=w848) -> ("Error Out"=w846:errorcluster, "Username Out"=w843:string)  [unwired: 7 in, 1 out]
            n398 = Index Array(array=w852, index=w851) -> (element=w849:string)
            n399 = Equal?(x=w849, y=w843) -> (x = y?=w845:bool)
            n400 = case shown="True" w845 {
              tunnel: [w861 w868] -> w847
              tunnel: w846 -> [w861 w867]
              tunnel: [State_-_Module_User_Management."Remove" State_-_Module_User_Management."Idle"] -> w844
              frame False {
              }
              frame True {
                n401 = call "Gen - Popup Single Button (Auto Close).vi"("Type"=enum16{"Error", "Info"}."Error", "Error in"=w867, "Auto Close? F"=TRUE, "Message in"="Cannot delete your account.", "Header"="Delete User") -> ("Error out"=w868:errorcluster)  [unwired: 5 in, 1 out]
              }
            }
          }
          frame "Remove" {
            # "Delete selected user."
            n402 = call "Gen - Popup Two Button.vi"("Type"=enum16{"Error", "Info"}."Info", "Error in"=w875, "Message in"="Are you sure to remove this user?", "Header"="Remove User") -> ("Error out"=w874:errorcluster, "Yes?"=w873:bool)  [unwired: 6 in]
            n403 = case shown="True" w873 {
              tunnel: w874 -> [w881 w892]
              tunnel: w877 -> [_ w888]
              tunnel: [w881 w886] -> w876
              tunnel: [State_-_Module_User_Management."Idle" State_-_Module_User_Management."Save User Authorization Info"] -> w870
              frame False {
              }
              frame True {
                n404 = Unbundle By Name(w888) -> ("Selected Row"=w889:i32)
                n405 = property on="User Information T" class="MCListbox (strict)"(error in=w892) -> (error out=w891:errorcluster, "ItemNames"=w890:string[][])  [unwired: 1 in, 1 out]
                n406 = Delete From Array(array=w890, index (row)=w889) -> (array with subset deleted=w885:string[][])  [unwired: 2 in, 1 out]
                n407 = property on="User Information T" class="MCListbox (strict)"(error in=w891, "ItemNames"=w885) -> (error out=w887:errorcluster)  [unwired: 1 in, 1 out]
                n408 = control-ref of="User Information"() -> (w884:refnum<vi>)
                n409 = call "User - Update User Table.vi"("Error In"=w887, "Max visible row"=7, "User Infor Ref"=w884, "User Information"=w885) -> ("Error Out"=w886:errorcluster)  [unwired: 6 in, 1 out]
              }
            }
          }
          frame "Block" {
            # "Block selected user. Block user cannot login."
            n410 = Unbundle By Name(w914) -> ("Selected Row"=w899:i32)
            n411 = property on="User Information" class="Arr"(error in=w905) -> (error out=w903:errorcluster, "Value"=w904:variant)  [unwired: 1 in, 1 out]
            n412 = Variant To Data(error in=w903, type=T3[] [] ("Array"), Variant=w904) -> (data=w900:T3[], error out=w902:errorcluster)
            n413 = Index Array(array=w900, index=w899) -> (element=w898:T3)
            n414 = Unbundle By Name(w898) -> ("Status"=w897:bool)
            n415 = Select(t="Block" ("new element/subarray"), s=w897, f="Unblock") -> (s? t:f=w894:string)
            n416 = property on="User Information T" class="MCListbox (strict)"(error in=w902) -> (error out=w917:errorcluster, "ItemNames"=w916:string[][])  [unwired: 1 in, 1 out]
            n417 = To Long Integer(number=Header_-_User_Management."Status" ("Header - User Management")) -> (32bit integer=w910:i32)
            n418 = Replace Array Subset(array=w916, new element=w894, index (row)=w899, index (col)=w910) -> (w906:string[][])
            n419 = property on="User Information T" class="MCListbox (strict)"(error in=w917, "ItemNames"=w906) -> (error out=w909:errorcluster)  [unwired: 1 in, 1 out]
            n420 = control-ref of="User Information"() -> (w907:refnum<vi>)
            n421 = call "User - Update User Table.vi"("Error In"=w909, "Max visible row"=7, "User Infor Ref"=w907, "User Information"=w906) -> ("Error Out"=w908:errorcluster)  [unwired: 6 in, 1 out]
            n422 = Bundle By Name(cluster=w914, "Selected Row"=-1 ("Row Clicked")) -> (w913:T8)
          }
          frame "Add Config Access Page" {
            n423 = property on="Manage: All Page" class="LstBox (strict)"(error in=w941) -> (error out=w947:errorcluster, "Item Names"=w926:string[], "Value"=w943:i32)  [unwired: 1 in, 1 out]
            n424 = Index Array(array=w926, index=w943) -> (element=w942:string)
            n425 = property on="Manage: Accessible Page" class="LstBox (strict)"(error in=w947) -> (error out=w928:errorcluster, "Item Names"=w946:string[])  [unwired: 1 in, 1 out]
            n426 = Insert Into Array(array=w946, new element=w942) -> (w945:string[])  [unwired: 1 in]
            n427 = call "Remove Duplicates From 1D Array.vim"("array"=w945) -> ("array with duplicates removed"=w944:string[])  [unwired: 10 in]
            n428 = Sort 1D Array(array=w944) -> (sorted array=w940:string[])
            n429 = call "Gen - System Config.vi"() -> ("Data Out"=w927:T18)  [unwired: 11 in]
            n430 = call "Gen - Remove Empty String Array.vi"("Data Array"=w940) -> ("Data Out"=w925:string[])  [unwired: 10 in]
            n431 = Unbundle By Name(w927) -> ("Page Module"=w924:string[], "Button.Text"=w923:string[])
            n432 = property on="Manage: Accessible Page" class="LstBox (strict)"(error in=w928, "Item Names"=w925) -> (error out=w921:errorcluster)  [unwired: 1 in, 1 out]
            n433 = call "User - Filter List.vi"("Error In"=w921, "Data to Search"=w925, "Search From"=w923, "All List"=w924) -> ("Error Out"=w920:errorcluster, "Data Out"=w922:string[])  [unwired: 6 in]
            n434 = call <vilib>:"1D String Array to Delimited String.vi"("delimiter"=",", "string array"=w922) -> ("delimited string"=w931:string)  [unwired: 9 in]
            n435 = property on="Manage: Access Level" class="CmbBox"(error in=w920) -> (error out=w935:errorcluster, "Value"=w936:string)  [unwired: 1 in, 1 out]
            n436 = property on="Header - User Access Level" class="Enum (strict)"(error in=w935) -> (error out=w938:errorcluster, "Strings []"=w937:string[])  [unwired: 1 in, 1 out]
            n437 = property on="Access Page T" class="LstBox (strict)"(error in=w938) -> (error out=w934:errorcluster, "Item Names"=w939:string[])  [unwired: 1 in, 1 out]
            n438 = Search 1D Array(1D array=w937, element=w936) -> (index of element=w932:i32)  [unwired: 1 in]
            n439 = Replace Array Subset(array=w939, new element=w931, index=w932) -> (w930:string[])
            n440 = property on="Access Page T" class="LstBox (strict)"(error in=w934, "Item Names"=w930) -> (error out=w933:errorcluster)  [unwired: 1 in, 1 out]
          }
          frame "Remove Config Access Page" {
            # "#Todo add into table"
            n441 = property on="Manage: Accessible Page" class="LstBox (strict)"(error in=w971) -> (error out=w957:errorcluster, "Item Names"=w973:string[], "Value"=w972:i32)  [unwired: 1 in, 1 out]
            n442 = call "Gen - System Config.vi"() -> ("Data Out"=w956:T18)  [unwired: 11 in]
            n443 = Unbundle By Name(w956) -> ("Page Module"=w955:string[], "Button.Text"=w954:string[])
            n444 = Delete From Array(array=w973, index=w972) -> (array with subset deleted=w962:string[])  [unwired: 1 in, 1 out]
            n445 = call "Gen - Remove Empty String Array.vi"("Data Array"=w962) -> ("Data Out"=w953:string[])  [unwired: 10 in]
            n446 = for {
              tunnel: w953 -> [w981] mode=indexing
              tunnel: w955 -> [w979]
              tunnel: w954 -> [w982]
              tunnel: [w978] -> w952 mode=indexing
              n447 = Search 1D Array(1D array=w982, element=w981) -> (index of element=w980:i32)  [unwired: 1 in]
              n448 = Index Array(array=w979, index=w980) -> (element=w978:string)
            }
            n449 = property on="Manage: Accessible Page" class="LstBox (strict)"(error in=w957, "Item Names"=w953) -> (error out=w964:errorcluster)  [unwired: 1 in, 1 out]
            n450 = call <vilib>:"1D String Array to Delimited String.vi"("delimiter"=",", "string array"=w952) -> ("delimited string"=w959:string)  [unwired: 9 in]
            n451 = property on="Manage: Access Level" class="CmbBox"(error in=w964) -> (error out=w967:errorcluster, "Value"=w968:string)  [unwired: 1 in, 1 out]
            n452 = property on="Header - User Access Level" class="Enum (strict)"(error in=w967) -> (error out=w970:errorcluster, "Strings []"=w969:string[])  [unwired: 1 in, 1 out]
            n453 = property on="Access Page T" class="LstBox (strict)"(error in=w970) -> (error out=w966:errorcluster, "Item Names"=w960:string[])  [unwired: 1 in, 1 out]
            n454 = Search 1D Array(1D array=w969, element=w968) -> (index of element=w961:i32)  [unwired: 1 in]
            n455 = Replace Array Subset(array=w960, new element=w959, index=w961) -> (w965:string[])
            n456 = property on="Access Page T" class="LstBox (strict)"(error in=w966, "Item Names"=w965) -> (error out=w963:errorcluster)  [unwired: 1 in, 1 out]
          }
          frame "Update Config User Access" {
            n457 = property on="Manage: Access Level" class="CmbBox"(error in=w995) -> (error out=w994:errorcluster, "Value"=w997:string)  [unwired: 1 in, 1 out]
            n458 = property on="Header - User Access Level" class="Enum (strict)"(error in=w994) -> (error out=w999:errorcluster, "Strings []"=w998:string[])  [unwired: 1 in, 1 out]
            n459 = call "Gen - System Config.vi"() -> ("Data Out"=w991:T18)  [unwired: 11 in]
            n460 = Unbundle By Name(w991) -> ("Button.Text"=w989:string[], "Page Module"=w990:string[])
            n461 = property on="Access Page T" class="LstBox (strict)"(error in=w999) -> (error out=w988:errorcluster, "Item Names"=w986:string[])  [unwired: 1 in, 1 out]
            n462 = Search 1D Array(1D array=w998, element=w997) -> (index of element=w996:i32)  [unwired: 1 in]
            n463 = Index Array(array=w986, index=w996) -> (element=w993:string)
            n464 = call <vilib>:"Delimited String to 1D String Array.vi"("delimiter"=",", "delimited string"=w993) -> ("string array"=w985:string[])  [unwired: 9 in]
            n465 = call "User - Filter List.vi"("Error In"=w988, "Data to Search"=w985, "Search From"=w990, "All List"=w989) -> ("Error Out"=w987:errorcluster, "Data Out"=w984:string[])  [unwired: 6 in]
            n466 = call "Gen - Remove Empty String Array.vi"("Data Array"=w984) -> ("Data Out"=w983:string[])  [unwired: 10 in]
            n467 = property on="Manage: Accessible Page" class="LstBox (strict)"(error in=w987, "Item Names"=w983) -> (error out=w1000:errorcluster)  [unwired: 1 in, 1 out]
          }
          frame "Save Config Access Page" {
            n468 = Unbundle By Name(w1005) -> ("Path User Access"=w1012:path)
            n469 = property on="Access Page T" class="LstBox (strict)"(error in=w1006) -> (error out=w1009:errorcluster, "Item Names"=w1010:string[])  [unwired: 1 in, 1 out]
            n470 = To Variant(anything=w1010) -> (Variant=w1011:variant)
            n471 = call "aFGV - Binary File.vi"("State"=enum16{"Read", "Write"}."Write", "Error In"=w1009, "Path"=w1012, "Data in"=w1011) -> ("Error Out"=w1007:errorcluster)  [unwired: 6 in, 1 out]
          }
          frame "Save Password Settg" {
            n472 = property on="User Information T" class="MCListbox (strict)"(error in=w1020, "Value"=-1 ("Multicolumn Listbox")) -> (error out=w1019:errorcluster)  [unwired: 1 in, 1 out]
            n473 = disable-structure shown="Disabled" {
              disable-tunnel: [w1037 w1051] -> w1027
              disable-tunnel: [w1036 FALSE ("cancelled")] -> w1026
              disable-tunnel: [w1035 w1052] -> w1025
              disable-tunnel: w1019 -> [w1029 w1052]
              disable-tunnel: w1016 -> [_ w1053]
              frame Disabled {
                n474 = call "Gen - File Directory.vi"("File Dir"=State_-_Directory."Password", "Error In"=w1029) -> ("error out"=w1031:errorcluster, "Application Directory"=w1028:path)  [unwired: 7 in, 1 out]
                n475 = call <vilib>:"Check if File or Folder Exists.vi"("error in (no error)"=w1031, "path"=w1028) -> ("error out"=w1034:errorcluster, "file or folder exists?"=w1033:bool, "dup path"=w1032:path)  [unwired: 7 in]
                n476 = case shown="False" w1033 {
                  selector: w1033 -> [_ w1047]
                  tunnel: [w1045 w1049] -> w1037
                  tunnel: [w1044 w1046] -> w1036
                  tunnel: [w1040 w1048] -> w1035
                  tunnel: w1034 -> [w1039 w1048]
                  tunnel: w1032 -> [_ w1049]
                  frame False {
                    n477 = call <vilib>:"Dflt Data Dir.vi"() -> ("App:Default Data Directory"=w1043:path)
                    n478 = feedback #1(w1043) -> (w1042:path)
                    n479 = call "File Dialog4"("start path"=w1042, "prompt"="Please specify the path to the Password Setting file..." ("pattern label"), "error in"=w1039, "pattern label"=".Pass") -> ("selected path"=w1045:path, "cancelled"=w1044:bool, "error out"=w1040:errorcluster)  [unwired: 8 in, 1 out]
                    n480 = feedback-in #1(w1045) -> ()
                  }
                  frame True {
                    n481 = Not(x=w1047) -> (.not. x?=w1046:bool)
                  }
                }
              }
              frame Enabled {
                n482 = Unbundle By Name(w1053) -> ("Path User Access"=w1051:path)
              }
            }
            n483 = Unbundle By Name(w1016) -> ("Password Setting"=w1018:T7)
            n484 = case shown="False" w1026 {
              tunnel: [w1055 w1063] -> w1024
              tunnel: w1025 -> [w1062 w1064]
              tunnel: w1027 -> [w1061 _]
              tunnel: w1018 -> [w1054 _]
              frame False {
                n485 = Open/Create/Replace File(file path (use dialog)=w1061, error in=w1062, operation (0:open)=T17."open or create") -> (refnum out=w1060:refnum<file>, error out=w1056:errorcluster)  [unwired: 3 in, 1 out]
                n486 = Write to Binary File(file (use dialog)=w1060, data=w1054, error in=w1056) -> (refnum out=w1058:refnum<file>, error out=w1059:errorcluster)  [unwired: 3 in, 1 out]
                n487 = Close File(refnum=w1058, error in=w1059) -> (error out=w1055:errorcluster)  [unwired: 1 out]
              }
              frame True {
                n488 = call <vilib>:"Clear Errors.vi"("error in (no error)"=w1064) -> ("error out"=w1063:errorcluster)  [unwired: 5 in, 1 out]
              }
            }
          }
          frame "Exit" {
            n489 = Unregister For Events(event registration refnum=w1066, error in=w1070) -> (error out=w1067:errorcluster)
          }
        }
      }
      frame Error {
        n490 = call <vilib>:"Clear Errors.vi"("error in (no error)"=w1073) -> ("error out"=w1075:errorcluster)  [unwired: 5 in, 1 out]
        n491 = call "Gen - Get Application Kind.vi"("Error In"=w1075) -> ("Application:Kind"=w1074:T24)  [unwired: 9 in, 1 out]
        n492 = case shown="\"Run Time System\"" w1074 {
          tunnel: [w1080 w1087 w1091] -> w1072
          tunnel: w1073 -> [w1080 w1083 w1089]
          tunnel: w1071 -> [_ w1084 _]
          frame "invalid app kind", Default {
          }
          frame "Run Time System" {
            n493 = Format Into String(error in=w1083, w1084) -> (resulting string=w1081:string, error out=w1082:errorcluster)  [unwired: 2 in]
            n494 = control-ref of="This VI"() -> (w1085:refnum<vi>)
            n495 = call "eFGV - Generated Error.vi"("eFGV States"=State_-_eFGV."Write", "Error In"=w1082, "State"=w1081, "This VI"=w1085) -> ("Error Out"=w1087:errorcluster)  [unwired: 6 in, 1 out]
          }
          frame "Development System" {
            n496 = call <vilib>:"Simple Error Handler.vi"("error in (no error)"=w1089) -> ("error?"=w1088:bool, "error out"=w1090:errorcluster)  [unwired: 4 in, 3 out]
            n497 = case shown="False" w1088 {
              tunnel: [w1092 w1094] -> w1091
              tunnel: w1090 -> [w1092 w1093]
              frame False {
              }
              frame True {
                n498 = call <vilib>:"Clear Errors.vi"("error in (no error)"=w1093) -> ("error out"=w1094:errorcluster)  [unwired: 5 in, 1 out]
              }
            }
          }
        }
      }
    }
    n499 = Wait (ms)(milliseconds to wait=u32 100) -> ()  [unwired: 1 out]
  }
  n500 = disable-structure shown="Enabled" {
    frame Disabled {
      n501 = Unbundle By Name() -> (w1095:T8, "User Information.All"=w1098)
      n502 = property on="Filter:" class="CmbBox"() -> (error out=w1097:errorcluster, "Strings[]"=w1099:string[], "Value"=w1100:string)  [unwired: 2 in, 1 out]
      n503 = Search 1D Array(1D array=w1099, element=w1100) -> (index of element=w1101:i32)  [unwired: 1 in]
      n504 = Decrement(x=w1101) -> (x-1=w1103:i32)
      n505 = Greater Or Equal To 0?(x=w1103) -> (x >= 0?=w1102:bool)
      n506 = case shown="True" w1102 {
        tunnel: [w1106 w1112] -> w1096
        tunnel: w1097 -> [w1106 w1111]
        tunnel: w1098 -> [w1107 w1110]
        tunnel: w1103 -> [_ w1109]
        tunnel: [w1107 w1108] -> w1105
        frame False {
        }
        frame True {
          n507 = for {
            tunnel: w1111 -> [w1118]
            tunnel: [w1118] -> w1112
            tunnel: w1110 -> [w1115]
            tunnel: w1109 -> [w1116]
            tunnel: [w1115] -> w1108 mode=indexing if=w1114
            n508 = Unbundle By Name(w1115) -> ("Access Level"=w1117)
            n509 = To Unsigned Word Integer(number=w1116) -> (unsigned 16bit integer=w1113:u16)
            n510 = Equal?(x=w1117, y=w1113) -> (x = y?=w1114:bool)
          }
        }
      }
      n511 = Bundle By Name(cluster=w1095, "Filtered"=w1105) -> (w1104:cluster{})
    }
    frame Disabled {
      n512 = property on="Config: Accessible Page" class="LstBox (strict)"() -> (error in=w1121:errorcluster, error out=w1122:errorcluster, "Item Names"=w1123:string[], "Value"=w1124:i32)  [unwired: 1 in, 1 out]
      n513 = Index Array(array=w1123, index=w1124) -> (element=w1125:string)
      n514 = property on="Config: Access Level" class="CmbBox"(error in=w1122) -> (error out=w1120:errorcluster, "Value"=w1119:string)  [unwired: 1 in, 1 out]
      n515 = case shown="\"Admin\"" w1119 {
        tunnel: [w1129 w1141] -> _
        tunnel: w1120 -> [w1130 w1141]
        tunnel: w1125 -> [w1132 _]
        tunnel: [w1128 State_-_Module_User_Management."Remove User Access Page"] -> w1126
        frame "Admin" {
          n516 = Equal?(x="USER", y=w1132) -> (x = y?=w1127:bool)
          n517 = case shown="True" w1127 {
            tunnel: w1130 -> [w1133 w1139]
            tunnel: [w1133 w1138] -> w1129
            tunnel: [State_-_Module_User_Management."Remove User Access Page" State_-_Module_User_Management."Idle"] -> w1128
            frame False {
            }
            frame True {
              n518 = call "Gen - Popup Single Button (Auto Close).vi"("Error in"=w1139, "Message in"="As an Admin, you cannot delete an access to this page.", "Header"="Delete Access Page") -> ("Error out"=w1138:errorcluster)  [unwired: 7 in, 1 out]
            }
          }
        }
        frame "Manager, Engineer, Technician", Default {
        }
      }
    }
    frame Enabled {
    }
  }
